vi "cDLTS measurement.vi"(5 "Session properties":T2, 7 "Workspace":path, 8 "Error In":errorcluster, 9 "myDLTS file path":path=path "", 10 "cDLTS measurement":T22={"Name"="", "Comment"="", "Time"=timestamp(0 s since 1904-01-01), "Folder"=path "", "DLTS properties"={"Tstart"=100.0, "Instant start"=FALSE, "Tstop"=350.0, "T rate"=0.016666666666666666, "Test signal"=0.1, "Test frequency"=100000.0, "Bandwidth"=0.0, "Averaging"=5.0, "Vbias"=-5.0, "Vpulse"=-1.0, "pulse length"=0.1, "Pulse 2"=FALSE, "Vpulse 2"=0.0, "pulse length 2"=0.0, "I range"=-2.0, "V range"=10.0, "Emission rate"=[10.0], "Sampling rate"=107000.0, "Acq. delay"=0.0, "Filter order"=0, "Equivalent circuit model"=0}, "GUID"=""} {"DLTS properties"."Equivalent circuit model" items=["Rp || Cp", "Rs + Cs", "Rs + Ls", "G B", "D Cs", "Q Cs", "D Ls", "Q Ls", "Rp || Lp", "D Cp"]; "DLTS properties"."Filter order" min=0 max=8 step=1; "DLTS properties"."Sampling rate" items=["13k"=13392.857422, "27k"=26785.714844, "54k"=53571.429687, "107k"=107142.859375]; "DLTS properties"."V range" items=["10mV"=0.01, "100mV"=0.1, "1V"=1.0, "10V"=10.0]; "DLTS properties"."I range" items=["10mV"=0.01, "100mV"=0.1, "1V"=1.0, "10V"=10.0]}, 11 "Loop data":T3={"Persistent"={"Last file"=path "", "Last user"="", "Users"=[]}, "Temp handle"={"Connected"=FALSE, "Temp ctrl"={"Gain (P)"=0.0, "Reset (I)"=0.0, "Rate (D)"=0.0, "Stabilization rate"=0.0, "Stabilization delta"=0.0, "Type"=enum."Lake Shore 325", "Custom temp ctrl"={"VISA resource name"=""}, "Lakeshore 325"={"VISA name"="", "Loop"=0, "Heater Range"=1, "Heater Resistance"=0, "Sample sensor"=0, "Fast sensor"=0, "Slow sensor"=0}, "Lakeshore 331"={"VISA name"="", "Loop"=1, "Heater Range"=0, "Sample sensor"=0, "Fast sensor"=0, "Slow sensor"=0}, "Lakeshore 332"={"VISA name"="", "Loop"=1, "Heater Range"=0, "Sample sensor"=0, "Fast sensor"=0, "Slow sensor"=0}, "Lakeshore 335"={"VISA name"="", "Loop"=1, "Sample sensor"=0, "Fast sensor"=0, "Slow sensor"=0, "Heater Range"=0, "Output mode"=enum."Off"}, "Lakeshore 336"={"VISA name"="", "Loop"=1, "Output mode"=enum."Off", "Max current"=1.0, "Heater resistance"=1, "Sample sensor"=1, "Slow sensor"=1, "Fast sensor"=1}}}, "Paths"={"Manual"=path "", "Settings"=path "", "Persistent"=path "", "Work dir."=path ""}, "Settings"={"MFIA"={"Address"="", "Use compensation"=TRUE, "Shut down gracefully"=FALSE}, "Temp ctrl"={"Gain (P)"=0.0, "Reset (I)"=0.0, "Rate (D)"=0.0, "Stabilization rate"=0.0, "Stabilization delta"=0.0, "Type"=enum."Lake Shore 325", "Custom temp ctrl"={"VISA resource name"=""}, "Lakeshore 325"={"VISA name"="", "Loop"=0, "Heater Range"=1, "Heater Resistance"=0, "Sample sensor"=0, "Fast sensor"=0, "Slow sensor"=0}, "Lakeshore 331"={"VISA name"="", "Loop"=1, "Heater Range"=0, "Sample sensor"=0, "Fast sensor"=0, "Slow sensor"=0}, "Lakeshore 332"={"VISA name"="", "Loop"=1, "Heater Range"=0, "Sample sensor"=0, "Fast sensor"=0, "Slow sensor"=0}, "Lakeshore 335"={"VISA name"="", "Loop"=1, "Sample sensor"=0, "Fast sensor"=0, "Slow sensor"=0, "Heater Range"=0, "Output mode"=enum."Off"}, "Lakeshore 336"={"VISA name"="", "Loop"=1, "Output mode"=enum."Off", "Max current"=1.0, "Heater resistance"=1, "Sample sensor"=1, "Slow sensor"=1, "Fast sensor"=1}}, "Source-meter"={"Type"=enum."Custom", "Custom source-meter"={"VISA resource name"=""}, "Keithley 2600"={"VISA name"="", "Ignore ID Query"=FALSE, "SMU"=enum."Channel A"}, "Keithley 2400 Series"={"VISA name"="", "Ignore ID Query"=FALSE}}, "Other"={"Enable OriginLab"=FALSE, "Reader mode"=FALSE, "Auto-save"=FALSE}, "Defaults"={"IV properties"={"T"=0.0, "Vstart"=-0.5, "Vstop"=0.5, "Vpoints"=10.0, "Settling"=0.01, "I limit"=0.1, "Log mapping"=FALSE, "Averaging"=0.0}, "CV properties"={"T"=0.0, "Vstart"=-0.5, "Vstop"=0.5, "Vpoints"=10.0, "Precision"=enum."Normal", "Test signal"=0.01, "Auto I range"=FALSE, "Test frequency"=100000.0, "I range"=-2.0, "V range"=10.0, "Log mapping"=FALSE, "Rel perm"=0.0, "Area"=0.0, "Equivalent circuit model"=0}, "DLTS properties"={"Tstart"=0.0, "Instant start"=FALSE, "Tstop"=0.0, "T rate"=0.0, "Test signal"=0.0, "Test frequency"=0.0, "Bandwidth"=0.0, "Averaging"=0.0, "Vbias"=0.0, "Vpulse"=0.0, "pulse length"=0.0, "Pulse 2"=FALSE, "Vpulse 2"=0.0, "pulse length 2"=0.0, "I range"=-2.0, "V range"=10.0, "Emission rate"=[], "Sampling rate"=0.0, "Acq. delay"=0.0, "Filter order"=0, "Equivalent circuit model"=0}, "LDLTS properties"={"T"=0.0, "Test signal"=0.0, "Test frequency"=0.0, "Bandwidth"=0.0, "Averaging"=0.0, "Vbias"=0.0, "Vpulse"=0.0, "pulse length"=0.0, "Pulse 2"=FALSE, "Vpulse 2"=0.0, "pulse length 2"=0.0, "I range"=-2.0, "V range"=10.0, "Sampling rate"=0.0, "Acq. delay"=0.0, "Sampling time"=0.0, "Filter order"=0, "Equivalent circuit model"=0}}}, "Software version"=0.0, "MFIA handle"={"ziHandle"={"handleValid"=FALSE, "Conn"=0, "Path Prefix"="", "Handle"=0, "Connected"=FALSE, "Clockbase(s)"=0.0}, "Selected device"="", "ziModHandle"={"handleValid"=FALSE, "Conn"=0, "ModHandle"=0, "moduleID"="", "Path Prefix"=""}}, "Source-meter handle"={"Connected"=FALSE, "Source-meter"={"Type"=enum."Custom", "Custom source-meter"={"VISA resource name"=""}, "Keithley 2600"={"VISA name"="", "Ignore ID Query"=FALSE, "SMU"=enum."Channel A"}, "Keithley 2400 Series"={"VISA name"="", "Ignore ID Query"=FALSE}}}} {"MFIA handle"."ziModHandle"."ModHandle" format="0x%08x"; "MFIA handle"."ziModHandle"."Conn" format="0x%08x"; "MFIA handle"."ziHandle"."Handle" format="0x%08x"; "MFIA handle"."ziHandle"."Conn" format="0x%08x"; "Settings"."Defaults"."LDLTS properties"."Equivalent circuit model" items=["Rp || Cp", "Rs + Cs", "Rs + Ls", "G B", "D Cs", "Q Cs", "D Ls", "Q Ls", "Rp || Lp", "D Cp"]; "Settings"."Defaults"."LDLTS properties"."Filter order" min=0 max=8 step=1; "Settings"."Defaults"."LDLTS properties"."Sampling rate" items=["13k"=13392.857422, "27k"=26785.714844, "54k"=53571.429687, "107k"=107142.859375]; "Settings"."Defaults"."LDLTS properties"."V range" items=["10mV"=0.01, "100mV"=0.1, "1V"=1.0, "10V"=10.0]; "Settings"."Defaults"."LDLTS properties"."I range" items=["100nA"=-7.0, "1µA"=-6.0, "10µA"=-5.0, "100µA"=-4.0, "1mA"=-3.0, "10mA"=-2.0]; "Settings"."Defaults"."DLTS properties"."Equivalent circuit model" items=["Rp || Cp", "Rs + Cs", "Rs + Ls", "G B", "D Cs", "Q Cs", "D Ls", "Q Ls", "Rp || Lp", "D Cp"]; "Settings"."Defaults"."DLTS properties"."Filter order" min=0 max=8 step=1; "Settings"."Defaults"."DLTS properties"."Sampling rate" items=["13k"=13392.857422, "27k"=26785.714844, "54k"=53571.429687, "107k"=107142.859375]; "Settings"."Defaults"."DLTS properties"."V range" items=["10mV"=0.01, "100mV"=0.1, "1V"=1.0, "10V"=10.0]; "Settings"."Defaults"."DLTS properties"."I range" items=["10mV"=0.01, "100mV"=0.1, "1V"=1.0, "10V"=10.0]; "Settings"."Defaults"."CV properties"."Equivalent circuit model" items=["Rp || Cp", "Rs + Cs", "Rs + Ls", "G B", "D Cs", "Q Cs", "D Ls", "Q Ls", "Rp || Lp", "D Cp"]; "Settings"."Defaults"."CV properties"."V range" items=["10mV"=0.01, "100mV"=0.1, "1V"=1.0, "10V"=10.0]; "Settings"."Defaults"."CV properties"."I range" items=["100nA"=-7.0, "1µA"=-6.0, "10µA"=-5.0, "100µA"=-4.0, "1mA"=-3.0, "10mA"=-2.0]; "Settings"."Defaults"."IV properties"."Settling" min=0.0 max=65535.0; "Settings"."Temp ctrl"."Lakeshore 336"."Fast sensor" items=["Sensor A", "Sensor B", "Sensor C", "Sensor D"]; "Settings"."Temp ctrl"."Lakeshore 336"."Slow sensor" items=["Sensor A", "Sensor B", "Sensor C", "Sensor D"]; "Settings"."Temp ctrl"."Lakeshore 336"."Sample sensor" items=["Sensor A", "Sensor B", "Sensor C", "Sensor D"]; "Settings"."Temp ctrl"."Lakeshore 336"."Heater resistance" items=["25 Ohm"=1, "50 Ohm"=2]; "Settings"."Temp ctrl"."Lakeshore 336"."Max current" items=["0.707 A"=0.0, "1 A"=1.0, "1.414 A"=1.414, "2 A"=2.0]; "Settings"."Temp ctrl"."Lakeshore 336"."Loop" items=["Output 1"=1, "Output 2"=2, "Output 3"=3, "Output 4"=4]; "Settings"."Temp ctrl"."Lakeshore 335"."Heater Range" items=["Off", "Low (On)", "Medium", "High"]; "Settings"."Temp ctrl"."Lakeshore 335"."Slow sensor" items=["A", "B"]; "Settings"."Temp ctrl"."Lakeshore 335"."Fast sensor" items=["A", "B"]; "Settings"."Temp ctrl"."Lakeshore 335"."Sample sensor" items=["A", "B"]; "Settings"."Temp ctrl"."Lakeshore 335"."Loop" items=["Loop 1"=1, "Loop 2"=2]; "Settings"."Temp ctrl"."Lakeshore 332"."Slow sensor" items=["A", "B"]; "Settings"."Temp ctrl"."Lakeshore 332"."Fast sensor" items=["A", "B"]; "Settings"."Temp ctrl"."Lakeshore 332"."Sample sensor" items=["A", "B"]; "Settings"."Temp ctrl"."Lakeshore 332"."Heater Range" items=["Off", "Low (0.5W)", "Med (5W)", "High (50W)"]; "Settings"."Temp ctrl"."Lakeshore 332"."Loop" items=["Loop 1", "Loop 2"]; "Settings"."Temp ctrl"."Lakeshore 331"."Slow sensor" items=["A", "B"]; "Settings"."Temp ctrl"."Lakeshore 331"."Fast sensor" items=["A", "B"]; "Settings"."Temp ctrl"."Lakeshore 331"."Sample sensor" items=["A", "B"]; "Settings"."Temp ctrl"."Lakeshore 331"."Heater Range" items=["Off", "Low (0.5W)", "Med (5W)", "High (50W)"]; "Settings"."Temp ctrl"."Lakeshore 331"."Loop" items=["Loop 1", "Loop 2"]; "Settings"."Temp ctrl"."Lakeshore 325"."Slow sensor" items=["A", "B"]; "Settings"."Temp ctrl"."Lakeshore 325"."Fast sensor" items=["A", "B"]; "Settings"."Temp ctrl"."Lakeshore 325"."Sample sensor" items=["A", "B"]; "Settings"."Temp ctrl"."Lakeshore 325"."Heater Resistance" items=["25 Ohm"=1, "50 Ohm"=2]; "Settings"."Temp ctrl"."Lakeshore 325"."Heater Range" items=["Off", "Low (loop 1) or On (loop 2)", "High (loop 1)"]; "Settings"."Temp ctrl"."Lakeshore 325"."Loop" items=["Loop 1"=1, "Loop 2"=2]; "Temp handle"."Temp ctrl"."Lakeshore 336"."Fast sensor" items=["Sensor A", "Sensor B", "Sensor C", "Sensor D"]; "Temp handle"."Temp ctrl"."Lakeshore 336"."Slow sensor" items=["Sensor A", "Sensor B", "Sensor C", "Sensor D"]; "Temp handle"."Temp ctrl"."Lakeshore 336"."Sample sensor" items=["Sensor A", "Sensor B", "Sensor C", "Sensor D"]; "Temp handle"."Temp ctrl"."Lakeshore 336"."Heater resistance" items=["25 Ohm"=1, "50 Ohm"=2]; "Temp handle"."Temp ctrl"."Lakeshore 336"."Max current" items=["0.707 A"=0.0, "1 A"=1.0, "1.414 A"=1.414, "2 A"=2.0]; "Temp handle"."Temp ctrl"."Lakeshore 336"."Loop" items=["Output 1"=1, "Output 2"=2, "Output 3"=3, "Output 4"=4]; "Temp handle"."Temp ctrl"."Lakeshore 335"."Heater Range" items=["Off", "Low (On)", "Medium", "High"]; "Temp handle"."Temp ctrl"."Lakeshore 335"."Slow sensor" items=["A", "B"]; "Temp handle"."Temp ctrl"."Lakeshore 335"."Fast sensor" items=["A", "B"]; "Temp handle"."Temp ctrl"."Lakeshore 335"."Sample sensor" items=["A", "B"]; "Temp handle"."Temp ctrl"."Lakeshore 335"."Loop" items=["Loop 1"=1, "Loop 2"=2]; "Temp handle"."Temp ctrl"."Lakeshore 332"."Slow sensor" items=["A", "B"]; "Temp handle"."Temp ctrl"."Lakeshore 332"."Fast sensor" items=["A", "B"]; "Temp handle"."Temp ctrl"."Lakeshore 332"."Sample sensor" items=["A", "B"]; "Temp handle"."Temp ctrl"."Lakeshore 332"."Heater Range" items=["Off", "Low (0.5W)", "Med (5W)", "High (50W)"]; "Temp handle"."Temp ctrl"."Lakeshore 332"."Loop" items=["Loop 1", "Loop 2"]; "Temp handle"."Temp ctrl"."Lakeshore 331"."Slow sensor" items=["A", "B"]; "Temp handle"."Temp ctrl"."Lakeshore 331"."Fast sensor" items=["A", "B"]; "Temp handle"."Temp ctrl"."Lakeshore 331"."Sample sensor" items=["A", "B"]; "Temp handle"."Temp ctrl"."Lakeshore 331"."Heater Range" items=["Off", "Low (0.5W)", "Med (5W)", "High (50W)"]; "Temp handle"."Temp ctrl"."Lakeshore 331"."Loop" items=["Loop 1", "Loop 2"]; "Temp handle"."Temp ctrl"."Lakeshore 325"."Slow sensor" items=["A", "B"]; "Temp handle"."Temp ctrl"."Lakeshore 325"."Fast sensor" items=["A", "B"]; "Temp handle"."Temp ctrl"."Lakeshore 325"."Sample sensor" items=["A", "B"]; "Temp handle"."Temp ctrl"."Lakeshore 325"."Heater Resistance" items=["25 Ohm"=1, "50 Ohm"=2]; "Temp handle"."Temp ctrl"."Lakeshore 325"."Heater Range" items=["Off", "Low (loop 1) or On (loop 2)", "High (loop 1)"]; "Temp handle"."Temp ctrl"."Lakeshore 325"."Loop" items=["Loop 1"=1, "Loop 2"=2]}) -> (0 "Error Out":errorcluster, 1 "Modified":bool, 2 "cDLTS measurement out":T22={"Name"="", "Comment"="", "Time"=timestamp(0 s since 1904-01-01), "Folder"=path "", "DLTS properties"={"Tstart"=0.0, "Instant start"=FALSE, "Tstop"=0.0, "T rate"=0.0, "Test signal"=0.0, "Test frequency"=0.0, "Bandwidth"=0.0, "Averaging"=0.0, "Vbias"=0.0, "Vpulse"=0.0, "pulse length"=0.0, "Pulse 2"=FALSE, "Vpulse 2"=0.0, "pulse length 2"=0.0, "I range"=-2.0, "V range"=10.0, "Emission rate"=[], "Sampling rate"=0.0, "Acq. delay"=0.0, "Filter order"=0, "Equivalent circuit model"=0}, "GUID"=""} {"DLTS properties"."Equivalent circuit model" items=["Rp || Cp", "Rs + Cs", "Rs + Ls", "G B", "D Cs", "Q Cs", "D Ls", "Q Ls", "Rp || Lp", "D Cp"]; "DLTS properties"."Filter order" min=0 max=8 step=1; "DLTS properties"."Sampling rate" items=["13k"=13392.857422, "27k"=26785.714844, "54k"=53571.429687, "107k"=107142.859375]; "DLTS properties"."V range" items=["10mV"=0.01, "100mV"=0.1, "1V"=1.0, "10V"=10.0]; "DLTS properties"."I range" items=["10mV"=0.01, "100mV"=0.1, "1V"=1.0, "10V"=10.0]}, 3 "Loop data out":T3={"Persistent"={"Last file"=path "", "Last user"="", "Users"=[]}, "Temp handle"={"Connected"=FALSE, "Temp ctrl"={"Gain (P)"=0.0, "Reset (I)"=0.0, "Rate (D)"=0.0, "Stabilization rate"=0.0, "Stabilization delta"=0.0, "Type"=enum."Lake Shore 325", "Custom temp ctrl"={"VISA resource name"=""}, "Lakeshore 325"={"VISA name"="", "Loop"=0, "Heater Range"=1, "Heater Resistance"=0, "Sample sensor"=0, "Fast sensor"=0, "Slow sensor"=0}, "Lakeshore 331"={"VISA name"="", "Loop"=1, "Heater Range"=0, "Sample sensor"=0, "Fast sensor"=0, "Slow sensor"=0}, "Lakeshore 332"={"VISA name"="", "Loop"=1, "Heater Range"=0, "Sample sensor"=0, "Fast sensor"=0, "Slow sensor"=0}, "Lakeshore 335"={"VISA name"="", "Loop"=1, "Sample sensor"=0, "Fast sensor"=0, "Slow sensor"=0, "Heater Range"=0, "Output mode"=enum."Off"}, "Lakeshore 336"={"VISA name"="", "Loop"=1, "Output mode"=enum."Off", "Max current"=1.0, "Heater resistance"=1, "Sample sensor"=1, "Slow sensor"=1, "Fast sensor"=1}}}, "Paths"={"Manual"=path "", "Settings"=path "", "Persistent"=path "", "Work dir."=path ""}, "Settings"={"MFIA"={"Address"="", "Use compensation"=TRUE, "Shut down gracefully"=FALSE}, "Temp ctrl"={"Gain (P)"=0.0, "Reset (I)"=0.0, "Rate (D)"=0.0, "Stabilization rate"=0.0, "Stabilization delta"=0.0, "Type"=enum."Lake Shore 325", "Custom temp ctrl"={"VISA resource name"=""}, "Lakeshore 325"={"VISA name"="", "Loop"=0, "Heater Range"=1, "Heater Resistance"=0, "Sample sensor"=0, "Fast sensor"=0, "Slow sensor"=0}, "Lakeshore 331"={"VISA name"="", "Loop"=1, "Heater Range"=0, "Sample sensor"=0, "Fast sensor"=0, "Slow sensor"=0}, "Lakeshore 332"={"VISA name"="", "Loop"=1, "Heater Range"=0, "Sample sensor"=0, "Fast sensor"=0, "Slow sensor"=0}, "Lakeshore 335"={"VISA name"="", "Loop"=1, "Sample sensor"=0, "Fast sensor"=0, "Slow sensor"=0, "Heater Range"=0, "Output mode"=enum."Off"}, "Lakeshore 336"={"VISA name"="", "Loop"=1, "Output mode"=enum."Off", "Max current"=1.0, "Heater resistance"=1, "Sample sensor"=1, "Slow sensor"=1, "Fast sensor"=1}}, "Source-meter"={"Type"=enum."Custom", "Custom source-meter"={"VISA resource name"=""}, "Keithley 2600"={"VISA name"="", "Ignore ID Query"=FALSE, "SMU"=enum."Channel A"}, "Keithley 2400 Series"={"VISA name"="", "Ignore ID Query"=FALSE}}, "Other"={"Enable OriginLab"=FALSE, "Reader mode"=FALSE, "Auto-save"=FALSE}, "Defaults"={"IV properties"={"T"=0.0, "Vstart"=-0.5, "Vstop"=0.5, "Vpoints"=10.0, "Settling"=0.01, "I limit"=0.1, "Log mapping"=FALSE, "Averaging"=0.0}, "CV properties"={"T"=0.0, "Vstart"=-0.5, "Vstop"=0.5, "Vpoints"=10.0, "Precision"=enum."Normal", "Test signal"=0.01, "Auto I range"=FALSE, "Test frequency"=100000.0, "I range"=-2.0, "V range"=10.0, "Log mapping"=FALSE, "Rel perm"=0.0, "Area"=0.0, "Equivalent circuit model"=0}, "DLTS properties"={"Tstart"=0.0, "Instant start"=FALSE, "Tstop"=0.0, "T rate"=0.0, "Test signal"=0.0, "Test frequency"=0.0, "Bandwidth"=0.0, "Averaging"=0.0, "Vbias"=0.0, "Vpulse"=0.0, "pulse length"=0.0, "Pulse 2"=FALSE, "Vpulse 2"=0.0, "pulse length 2"=0.0, "I range"=-2.0, "V range"=10.0, "Emission rate"=[], "Sampling rate"=0.0, "Acq. delay"=0.0, "Filter order"=0, "Equivalent circuit model"=0}, "LDLTS properties"={"T"=0.0, "Test signal"=0.0, "Test frequency"=0.0, "Bandwidth"=0.0, "Averaging"=0.0, "Vbias"=0.0, "Vpulse"=0.0, "pulse length"=0.0, "Pulse 2"=FALSE, "Vpulse 2"=0.0, "pulse length 2"=0.0, "I range"=-2.0, "V range"=10.0, "Sampling rate"=0.0, "Acq. delay"=0.0, "Sampling time"=0.0, "Filter order"=0, "Equivalent circuit model"=0}}}, "Software version"=0.0, "MFIA handle"={"ziHandle"={"handleValid"=FALSE, "Conn"=0, "Path Prefix"="", "Handle"=0, "Connected"=FALSE, "Clockbase(s)"=0.0}, "Selected device"="", "ziModHandle"={"handleValid"=FALSE, "Conn"=0, "ModHandle"=0, "moduleID"="", "Path Prefix"=""}}, "Source-meter handle"={"Connected"=FALSE, "Source-meter"={"Type"=enum."Custom", "Custom source-meter"={"VISA resource name"=""}, "Keithley 2600"={"VISA name"="", "Ignore ID Query"=FALSE, "SMU"=enum."Channel A"}, "Keithley 2400 Series"={"VISA name"="", "Ignore ID Query"=FALSE}}}} {"MFIA handle"."ziModHandle"."ModHandle" format="0x%08x"; "MFIA handle"."ziModHandle"."Conn" format="0x%08x"; "MFIA handle"."ziHandle"."Handle" format="0x%08x"; "MFIA handle"."ziHandle"."Conn" format="0x%08x"; "Settings"."Defaults"."LDLTS properties"."Equivalent circuit model" items=["Rp || Cp", "Rs + Cs", "Rs + Ls", "G B", "D Cs", "Q Cs", "D Ls", "Q Ls", "Rp || Lp", "D Cp"]; "Settings"."Defaults"."LDLTS properties"."Filter order" min=0 max=8 step=1; "Settings"."Defaults"."LDLTS properties"."Sampling rate" items=["13k"=13392.857422, "27k"=26785.714844, "54k"=53571.429687, "107k"=107142.859375]; "Settings"."Defaults"."LDLTS properties"."V range" items=["10mV"=0.01, "100mV"=0.1, "1V"=1.0, "10V"=10.0]; "Settings"."Defaults"."LDLTS properties"."I range" items=["100nA"=-7.0, "1µA"=-6.0, "10µA"=-5.0, "100µA"=-4.0, "1mA"=-3.0, "10mA"=-2.0]; "Settings"."Defaults"."DLTS properties"."Equivalent circuit model" items=["Rp || Cp", "Rs + Cs", "Rs + Ls", "G B", "D Cs", "Q Cs", "D Ls", "Q Ls", "Rp || Lp", "D Cp"]; "Settings"."Defaults"."DLTS properties"."Filter order" min=0 max=8 step=1; "Settings"."Defaults"."DLTS properties"."Sampling rate" items=["13k"=13392.857422, "27k"=26785.714844, "54k"=53571.429687, "107k"=107142.859375]; "Settings"."Defaults"."DLTS properties"."V range" items=["10mV"=0.01, "100mV"=0.1, "1V"=1.0, "10V"=10.0]; "Settings"."Defaults"."DLTS properties"."I range" items=["10mV"=0.01, "100mV"=0.1, "1V"=1.0, "10V"=10.0]; "Settings"."Defaults"."CV properties"."Equivalent circuit model" items=["Rp || Cp", "Rs + Cs", "Rs + Ls", "G B", "D Cs", "Q Cs", "D Ls", "Q Ls", "Rp || Lp", "D Cp"]; "Settings"."Defaults"."CV properties"."V range" items=["10mV"=0.01, "100mV"=0.1, "1V"=1.0, "10V"=10.0]; "Settings"."Defaults"."CV properties"."I range" items=["100nA"=-7.0, "1µA"=-6.0, "10µA"=-5.0, "100µA"=-4.0, "1mA"=-3.0, "10mA"=-2.0]; "Settings"."Defaults"."IV properties"."Settling" min=0.0 max=65535.0; "Settings"."Temp ctrl"."Lakeshore 336"."Fast sensor" items=["Sensor A", "Sensor B", "Sensor C", "Sensor D"]; "Settings"."Temp ctrl"."Lakeshore 336"."Slow sensor" items=["Sensor A", "Sensor B", "Sensor C", "Sensor D"]; "Settings"."Temp ctrl"."Lakeshore 336"."Sample sensor" items=["Sensor A", "Sensor B", "Sensor C", "Sensor D"]; "Settings"."Temp ctrl"."Lakeshore 336"."Heater resistance" items=["25 Ohm"=1, "50 Ohm"=2]; "Settings"."Temp ctrl"."Lakeshore 336"."Max current" items=["0.707 A"=0.0, "1 A"=1.0, "1.414 A"=1.414, "2 A"=2.0]; "Settings"."Temp ctrl"."Lakeshore 336"."Loop" items=["Output 1"=1, "Output 2"=2, "Output 3"=3, "Output 4"=4]; "Settings"."Temp ctrl"."Lakeshore 335"."Heater Range" items=["Off", "Low (On)", "Medium", "High"]; "Settings"."Temp ctrl"."Lakeshore 335"."Slow sensor" items=["A", "B"]; "Settings"."Temp ctrl"."Lakeshore 335"."Fast sensor" items=["A", "B"]; "Settings"."Temp ctrl"."Lakeshore 335"."Sample sensor" items=["A", "B"]; "Settings"."Temp ctrl"."Lakeshore 335"."Loop" items=["Loop 1"=1, "Loop 2"=2]; "Settings"."Temp ctrl"."Lakeshore 332"."Slow sensor" items=["A", "B"]; "Settings"."Temp ctrl"."Lakeshore 332"."Fast sensor" items=["A", "B"]; "Settings"."Temp ctrl"."Lakeshore 332"."Sample sensor" items=["A", "B"]; "Settings"."Temp ctrl"."Lakeshore 332"."Heater Range" items=["Off", "Low (0.5W)", "Med (5W)", "High (50W)"]; "Settings"."Temp ctrl"."Lakeshore 332"."Loop" items=["Loop 1", "Loop 2"]; "Settings"."Temp ctrl"."Lakeshore 331"."Slow sensor" items=["A", "B"]; "Settings"."Temp ctrl"."Lakeshore 331"."Fast sensor" items=["A", "B"]; "Settings"."Temp ctrl"."Lakeshore 331"."Sample sensor" items=["A", "B"]; "Settings"."Temp ctrl"."Lakeshore 331"."Heater Range" items=["Off", "Low (0.5W)", "Med (5W)", "High (50W)"]; "Settings"."Temp ctrl"."Lakeshore 331"."Loop" items=["Loop 1", "Loop 2"]; "Settings"."Temp ctrl"."Lakeshore 325"."Slow sensor" items=["A", "B"]; "Settings"."Temp ctrl"."Lakeshore 325"."Fast sensor" items=["A", "B"]; "Settings"."Temp ctrl"."Lakeshore 325"."Sample sensor" items=["A", "B"]; "Settings"."Temp ctrl"."Lakeshore 325"."Heater Resistance" items=["25 Ohm"=1, "50 Ohm"=2]; "Settings"."Temp ctrl"."Lakeshore 325"."Heater Range" items=["Off", "Low (loop 1) or On (loop 2)", "High (loop 1)"]; "Settings"."Temp ctrl"."Lakeshore 325"."Loop" items=["Loop 1"=1, "Loop 2"=2]; "Temp handle"."Temp ctrl"."Lakeshore 336"."Fast sensor" items=["Sensor A", "Sensor B", "Sensor C", "Sensor D"]; "Temp handle"."Temp ctrl"."Lakeshore 336"."Slow sensor" items=["Sensor A", "Sensor B", "Sensor C", "Sensor D"]; "Temp handle"."Temp ctrl"."Lakeshore 336"."Sample sensor" items=["Sensor A", "Sensor B", "Sensor C", "Sensor D"]; "Temp handle"."Temp ctrl"."Lakeshore 336"."Heater resistance" items=["25 Ohm"=1, "50 Ohm"=2]; "Temp handle"."Temp ctrl"."Lakeshore 336"."Max current" items=["0.707 A"=0.0, "1 A"=1.0, "1.414 A"=1.414, "2 A"=2.0]; "Temp handle"."Temp ctrl"."Lakeshore 336"."Loop" items=["Output 1"=1, "Output 2"=2, "Output 3"=3, "Output 4"=4]; "Temp handle"."Temp ctrl"."Lakeshore 335"."Heater Range" items=["Off", "Low (On)", "Medium", "High"]; "Temp handle"."Temp ctrl"."Lakeshore 335"."Slow sensor" items=["A", "B"]; "Temp handle"."Temp ctrl"."Lakeshore 335"."Fast sensor" items=["A", "B"]; "Temp handle"."Temp ctrl"."Lakeshore 335"."Sample sensor" items=["A", "B"]; "Temp handle"."Temp ctrl"."Lakeshore 335"."Loop" items=["Loop 1"=1, "Loop 2"=2]; "Temp handle"."Temp ctrl"."Lakeshore 332"."Slow sensor" items=["A", "B"]; "Temp handle"."Temp ctrl"."Lakeshore 332"."Fast sensor" items=["A", "B"]; "Temp handle"."Temp ctrl"."Lakeshore 332"."Sample sensor" items=["A", "B"]; "Temp handle"."Temp ctrl"."Lakeshore 332"."Heater Range" items=["Off", "Low (0.5W)", "Med (5W)", "High (50W)"]; "Temp handle"."Temp ctrl"."Lakeshore 332"."Loop" items=["Loop 1", "Loop 2"]; "Temp handle"."Temp ctrl"."Lakeshore 331"."Slow sensor" items=["A", "B"]; "Temp handle"."Temp ctrl"."Lakeshore 331"."Fast sensor" items=["A", "B"]; "Temp handle"."Temp ctrl"."Lakeshore 331"."Sample sensor" items=["A", "B"]; "Temp handle"."Temp ctrl"."Lakeshore 331"."Heater Range" items=["Off", "Low (0.5W)", "Med (5W)", "High (50W)"]; "Temp handle"."Temp ctrl"."Lakeshore 331"."Loop" items=["Loop 1", "Loop 2"]; "Temp handle"."Temp ctrl"."Lakeshore 325"."Slow sensor" items=["A", "B"]; "Temp handle"."Temp ctrl"."Lakeshore 325"."Fast sensor" items=["A", "B"]; "Temp handle"."Temp ctrl"."Lakeshore 325"."Sample sensor" items=["A", "B"]; "Temp handle"."Temp ctrl"."Lakeshore 325"."Heater Resistance" items=["25 Ohm"=1, "50 Ohm"=2]; "Temp handle"."Temp ctrl"."Lakeshore 325"."Heater Range" items=["Off", "Low (loop 1) or On (loop 2)", "High (loop 1)"]; "Temp handle"."Temp ctrl"."Lakeshore 325"."Loop" items=["Loop 1"=1, "Loop 2"=2]})   [LabVIEW 2019]
doc: "Handles conventional DLTS measurement, displays cDLTS GUI window"
uses:
  Type defs/Loop data Type Def.ctl
  Type defs/Persistent Type Def.ctl
  Type defs/Temp handle Type Def.ctl
  Type defs/Temp ctrl Type Def.ctl
  Custom devices/Custom temp ctrl settings.ctl
  Type defs/Paths Type Def.ctl
  Type defs/Settings Type Def.ctl
  Type defs/Imps Type Def.ctl
  Type defs/Source-meter Type Def.ctl
  Custom devices/Custom source-meter settings.ctl
  Type defs/Other settings Type Def.ctl
  Type defs/IV properties Type Def.ctl
  Type defs/CV properties Type Def.ctl
  Type defs/DLTS properties Type Def.ctl
  Type defs/LDLTS properties Type Def.ctl
  Type defs/MFIA handle Type Def.ctl
  <instrlib>/Zurich Instruments LabOne/Public/ziTypeHandle.ctl
  <instrlib>/Zurich Instruments LabOne/Public/Modules/ziTypeModHandle.ctl
  Type defs/Source-meter handle Type Def.ctl
  Type defs/cDLTS measurement Type Def.ctl
  Type defs/Session properties Type Def.ctl
  <vilib>/Utility/miscctls.llb/LVPointTypeDef.ctl
  <vilib>/Utility/error.llb/DialogType.ctl
  <vilib>/TaskbarProgressAPI/_TypeDefs/Progress State.ctl
  DLTS - timing calculation (time window) (SubVI).vi
  <instrlib>/Zurich Instruments LabOne/Public/Configure/ziSetValueDouble.vi
  Export single clipboard - cDLTS cluster.vi
  Export single dat - cDLTS cluster.vi
  Export Origin - cDLTS.vi
  DLTS - timing calculation (emission rates) (SubVI).vi
  <instrlib>/Zurich Instruments LabOne/Zurich Instruments LabOne.lvlib
  <vilib>/TaskbarProgressAPI/TaskbarProgressAPI.lvlib
panel:
  in  "Model":u16(ring) caption="Equivalent circuit model" items=["Rp || Cp", "Rs + Cs"]
  in  "Filter order":i32=8 caption="Numeric" min=1 max=8 step=1
  out "Filter rise time":dbl[unit]=10.0 caption="Numeric" min=0.1 max=100.0 format="%#_2p"
  in  "Folder":path
  in  "Enable post meas. T":bool caption="Enable"
  in  "Post meas. temp.":dbl[unit]=300.0 caption="Numeric" min=1.0 max=800.0 format="%#.0f"
  in  "Acquisition delay":dbl[unit]=1.0 caption="Numeric" min=0.0 max=1.0 step=1e-06 format="%#_6p"
  in  "2nd pulse":bool=TRUE caption="2 pulse mode:"
  in  "2nd pulse length":dbl[unit]=100.0 caption="2nd pulse duration" min=1e-06 max=100.0 format="%#_6p"
  in  "2nd pulse voltage":dbl[unit]=0.01 caption="Numeric" min=-10.0 max=10.0 format="%#_6p"
  in  "Sampling rate":dbl(ring)=107142.859375 caption="Ring" items=["13 kSa"=13392.857422, "27 kSa"=26785.714844, "54 kSa"=53571.429687, "107 kSa"=107142.859375]
  in  "Filter bandwidth":dbl[unit]=10000.0 caption="Numeric" min=100.0 max=100000.0 format="%#_6p"
  in  "Stop":bool
  out "Single transient capture duration":dbl[unit] caption="Numeric" format="%#.1p"
  out "No samples":dbl caption="Number of samples per transient" format="%#.0f"
  in  "Rate windows":dbl[unit][](array[numeric]) min=1.0 max=5000.0
  in  "Averaging":dbl=1.0 caption="Numeric" min=1.0 max=300.0 step=1.0
  in  "1st pulse length":dbl[unit]=100.0 caption="1st pulse duration" min=2.333e-07 max=1.0 format="%#.1p"
  in  "1st pulse voltage":dbl[unit]=0.01 caption="Numeric" min=-10.0 max=10.0 format="%#_6p"
  in  "Bias voltage":dbl[unit]=0.01 caption="Numeric" min=-10.0 max=10.0 format="%#_6p"
  in  "T rate":dbl[unit]=1.6666666666666667e-05 caption="Temperature change rate" min=1.6666666666666667e-05 max=1.6666666666666667 format="%#.1g"
  in  "Instant T start":bool=TRUE caption="Instant"
  in  "Stop temp.":dbl[unit]=1.0 caption="Numeric" min=1.0 max=800.0
  in  "Start temp.":dbl[unit]=1.0 caption="Numeric" min=1.0 max=800.0 format="%#.0f"
  in  "V range":dbl[unit](ring)=10.0 caption="Voltage range" items=["10mV"=0.01, "100mV"=0.1, "1V"=1.0, "10V"=10.0]
  in  "Test frequency":dbl[unit]=100000.0 caption="Numeric" min=10000.0 max=5000000000.0 format="%#_6p"
  in  "I range":dbl(ring)=-7.0 caption="Current range" items=["100nA"=-7.0, "1µA"=-6.0, "10µA"=-5.0, "100µA"=-4.0, "1mA"=-3.0, "10mA"=-2.0]
  in  "Measure":bool
  in  "Test signal":dbl[unit]=0.3 caption="Numeric" min=1e-06 max=1.0 format="%#_6p"
  in  "Setpoint":dbl[unit]=1.0 caption="Numeric" min=1.0 max=800.0
  out "Temperature":dbl[unit] caption="Numeric"
  out "Measurement info":string
  in  "Top Buttons":T1
  out "DLTS Signal Graph":cluster{"2D data":dbl[], "2D data":dbl[]}[](graph)
  out "Transient Graph":cluster{"t":dbl[], "Samples":dbl[]}(graph)
  out "Temp Chart":dbl(graph)=189.08
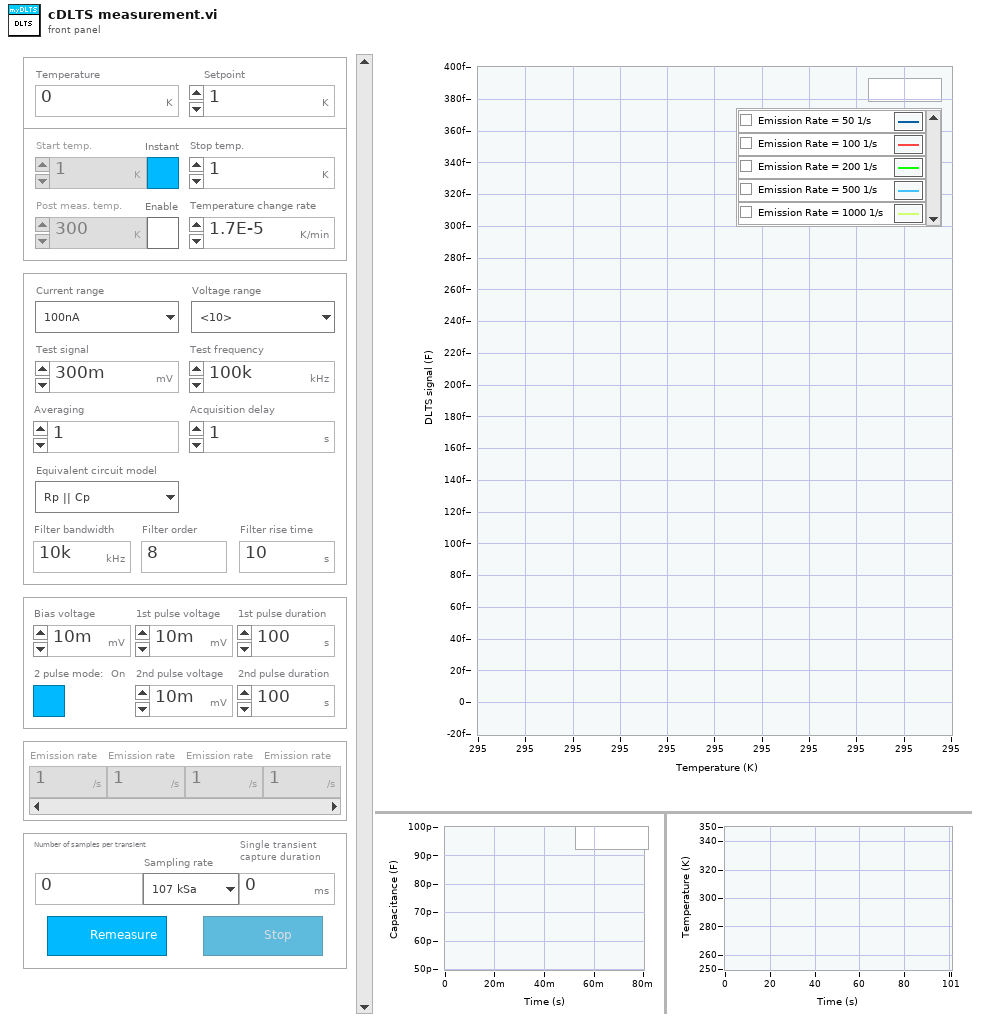
[diagram p1: front panel]
types:
  T1 = cluster{"Information":bool, "Help":bool, "Save Parameters":bool, "Export":bool}
  T2 = typedef "Session properties Type Def.ctl" = cluster{"Session name":string, "Comment":string, "User":string, "Software version":dbl, "Created":timestamp, "Modified":timestamp, "Binary":bool, "GUID":string}
  T3 = typedef "Loop data Type Def.ctl" = cluster{"Persistent":T4, "Temp handle":T5, "Paths":T8, "Settings":T9, "Software version":dbl, "MFIA handle":T18, "Source-meter handle":T21}
  T4 = typedef "Persistent Type Def.ctl" = cluster{"Last file":path, "Last user":string, "Users":cluster{"User":string, "Authors directory":path}[]}
  T5 = typedef "Temp handle Type Def.ctl" = cluster{"Connected":bool, "Temp ctrl":T6}
  T6 = typedef "Temp ctrl Type Def.ctl" = cluster{"Gain (P)":dbl, "Reset (I)":dbl, "Rate (D)":dbl, "Stabilization rate":dbl, "Stabilization delta":dbl, "Type":enum16{"Custom", "Lake Shore 325", "Lake Shore 331", "Lake Shore 332", "Lake Shore 335", "Lake Shore 336"}, "Custom temp ctrl":T7, "Lakeshore 325":cluster{"VISA name":refnum<visa-resource-name>, "Loop":u16, "Heater Range":u16, "Heater Resistance":u16, "Sample sensor":u16, "Fast sensor":u16, "Slow sensor":u16}, "Lakeshore 331":cluster{"VISA name":refnum<visa-resource-name>, "Loop":u16, "Heater Range":u16, "Sample sensor":u16, "Fast sensor":u16, "Slow sensor":u16}, "Lakeshore 332":cluster{"VISA name":refnum<visa-resource-name>, "Loop":u16, "Heater Range":u16, "Sample sensor":u16, "Fast sensor":u16, "Slow sensor":u16}, "Lakeshore 335":cluster{"VISA name":refnum<visa-resource-name>, "Loop":u16, "Sample sensor":u16, "Fast sensor":u16, "Slow sensor":u16, "Heater Range":u16, "Output mode":enum16{"Off", "Closed Loop PID", "Zone", "Open Loop", "Monitor Out", "Warmup Supply"}}, "Lakeshore 336":cluster{"VISA name":refnum<visa-resource-name>, "Loop":u16, "Output mode":enum16{"Off", "Closed Loop PID", "Zone", "Open Loop"}, "Max current":dbl, "Heater resistance":u16, "Sample sensor":u16, "Slow sensor":u16, "Fast sensor":u16}}
  T7 = typedef "Custom temp ctrl settings.ctl" = cluster{"VISA resource name":refnum<visa-resource-name>}
  T8 = typedef "Paths Type Def.ctl" = cluster{"Manual":path, "Settings":path, "Persistent":path, "Work dir.":path}
  T9 = typedef "Settings Type Def.ctl" = cluster{"MFIA":T10, "Temp ctrl":T6, "Source-meter":T11, "Other":T13, "Defaults":cluster{"IV properties":T14, "CV properties":T15, "DLTS properties":T16, "LDLTS properties":T17}}
  T10 = typedef "Imps Type Def.ctl" = cluster{"Address":string, "Use compensation":bool, "Shut down gracefully":bool}
  T11 = typedef "Source-meter Type Def.ctl" = cluster{"Type":enum16{"Custom", "Keithley 2600", "Keithley 2400 Series"}, "Custom source-meter":T12, "Keithley 2600":cluster{"VISA name":refnum<visa-resource-name>, "Ignore ID Query":bool, "SMU":enum16{"Channel A", "Channel B"}}, "Keithley 2400 Series":cluster{"VISA name":refnum<visa-resource-name>, "Ignore ID Query":bool}}
  T12 = typedef "Custom source-meter settings.ctl" = cluster{"VISA resource name":refnum<visa-resource-name>}
  T13 = typedef "Other settings Type Def.ctl" = cluster{"Enable OriginLab":bool, "Reader mode":bool, "Auto-save":bool}
  T14 = typedef "IV properties Type Def.ctl" = cluster{"T":dbl[unit], "Vstart":dbl[unit], "Vstop":dbl[unit], "Vpoints":dbl, "Settling":dbl[unit], "I limit":dbl[unit], "Log mapping":bool, "Averaging":dbl}
  T15 = typedef "CV properties Type Def.ctl" = cluster{"T":dbl[unit], "Vstart":dbl[unit], "Vstop":dbl[unit], "Vpoints":dbl, "Precision":enum16{"Low (Fast)", "Normal", "High (Slow)"}, "Test signal":dbl[unit], "Auto I range":bool, "Test frequency":dbl[unit], "I range":dbl, "V range":dbl[unit], "Log mapping":bool, "Rel perm":dbl, "Area":dbl[unit], "Equivalent circuit model":u16}
  T16 = typedef "DLTS properties Type Def.ctl" = cluster{"Tstart":dbl[unit], "Instant start":bool, "Tstop":dbl[unit], "T rate":dbl[unit], "Test signal":dbl[unit], "Test frequency":dbl[unit], "Bandwidth":dbl[unit], "Averaging":dbl, "Vbias":dbl[unit], "Vpulse":dbl[unit], "pulse length":dbl[unit], "Pulse 2":bool, "Vpulse 2":dbl[unit], "pulse length 2":dbl[unit], "I range":dbl, "V range":dbl[unit], "Emission rate":dbl[unit][], "Sampling rate":dbl[unit], "Acq. delay":dbl[unit], "Filter order":i32, "Equivalent circuit model":u16}
  T17 = typedef "LDLTS properties Type Def.ctl" = cluster{"T":dbl[unit], "Test signal":dbl[unit], "Test frequency":dbl[unit], "Bandwidth":dbl[unit], "Averaging":dbl, "Vbias":dbl[unit], "Vpulse":dbl[unit], "pulse length":dbl[unit], "Pulse 2":bool, "Vpulse 2":dbl[unit], "pulse length 2":dbl[unit], "I range":dbl, "V range":dbl[unit], "Sampling rate":dbl[unit], "Acq. delay":dbl[unit], "Sampling time":dbl[unit], "Filter order":i32, "Equivalent circuit model":u16}
  T18 = typedef "MFIA handle Type Def.ctl" = cluster{"ziHandle":T19, "Selected device":string, "ziModHandle":T20}
  T19 = typedef "Zurich Instruments LabOne.lvlib/ziTypeHandle.ctl" = cluster{"handleValid":bool, "Conn":u64, "Path Prefix":string, "Handle":u64, "Connected":bool, "Clockbase(s)":dbl}
  T20 = typedef "Zurich Instruments LabOne.lvlib/ziTypeModHandle.ctl" = cluster{"handleValid":bool, "Conn":u64, "ModHandle":u64, "moduleID":string, "Path Prefix":string}
  T21 = typedef "Source-meter handle Type Def.ctl" = cluster{"Connected":bool, "Source-meter":T11}
  T22 = typedef "cDLTS measurement Type Def.ctl" = cluster{"Name":string, "Comment":string, "Time":timestamp, "Folder":path, "DLTS properties":T16, "GUID":string}
  T23 = cluster{"Timestamps":ext[], "Temperatures":dbl[unit][]}
  T24 = cluster{"MFIA":bool, "Temperature controller":bool, "Source meter":bool}
  T25 = cluster{"Settings":T9, "DLTS properties":T16, "actual t_w":dbl[unit][], "R_peak":dbl[]}
  T26 = typedef "LVPointTypeDef.ctl" = cluster{"Horizontal":i16, "Vertical":i16}
  T27 = cluster{"Message":string, "C(t)":dbl[unit][], "t":dbl[unit][], "tau":dbl[unit][], "T":dbl[unit], "actual t_w":dbl[unit][], "R_peak":dbl[]}
  T28 = enum8{"Enabled", "Disabled", "Disabled and Grayed Out"}
  T29 = typedef "Semaphore RefNum" = refnum<k1>
  T30 = typedef "DialogType.ctl" = u16
  T31 = typedef "TaskbarProgressAPI.lvlib/Progress State.ctl" = i32
  T32 = cluster{"t":dbl[], "Capacitance transient":dbl[]}
  T33 = cluster{"Clipboard":bool, "dat":bool, "iso":bool, "Origin":bool, "Excel":bool}
  T34 = cluster{"T_s 50%":dbl[unit], "T_s 1-1/e":dbl[unit], "T_s 90%":dbl[unit], "T_s 95%":dbl[unit], "T_s 99%":dbl[unit]}
  T35 = enum16{"Canceled", "Clipboard", "Dat", "Iso", "Origin", "Excel"}
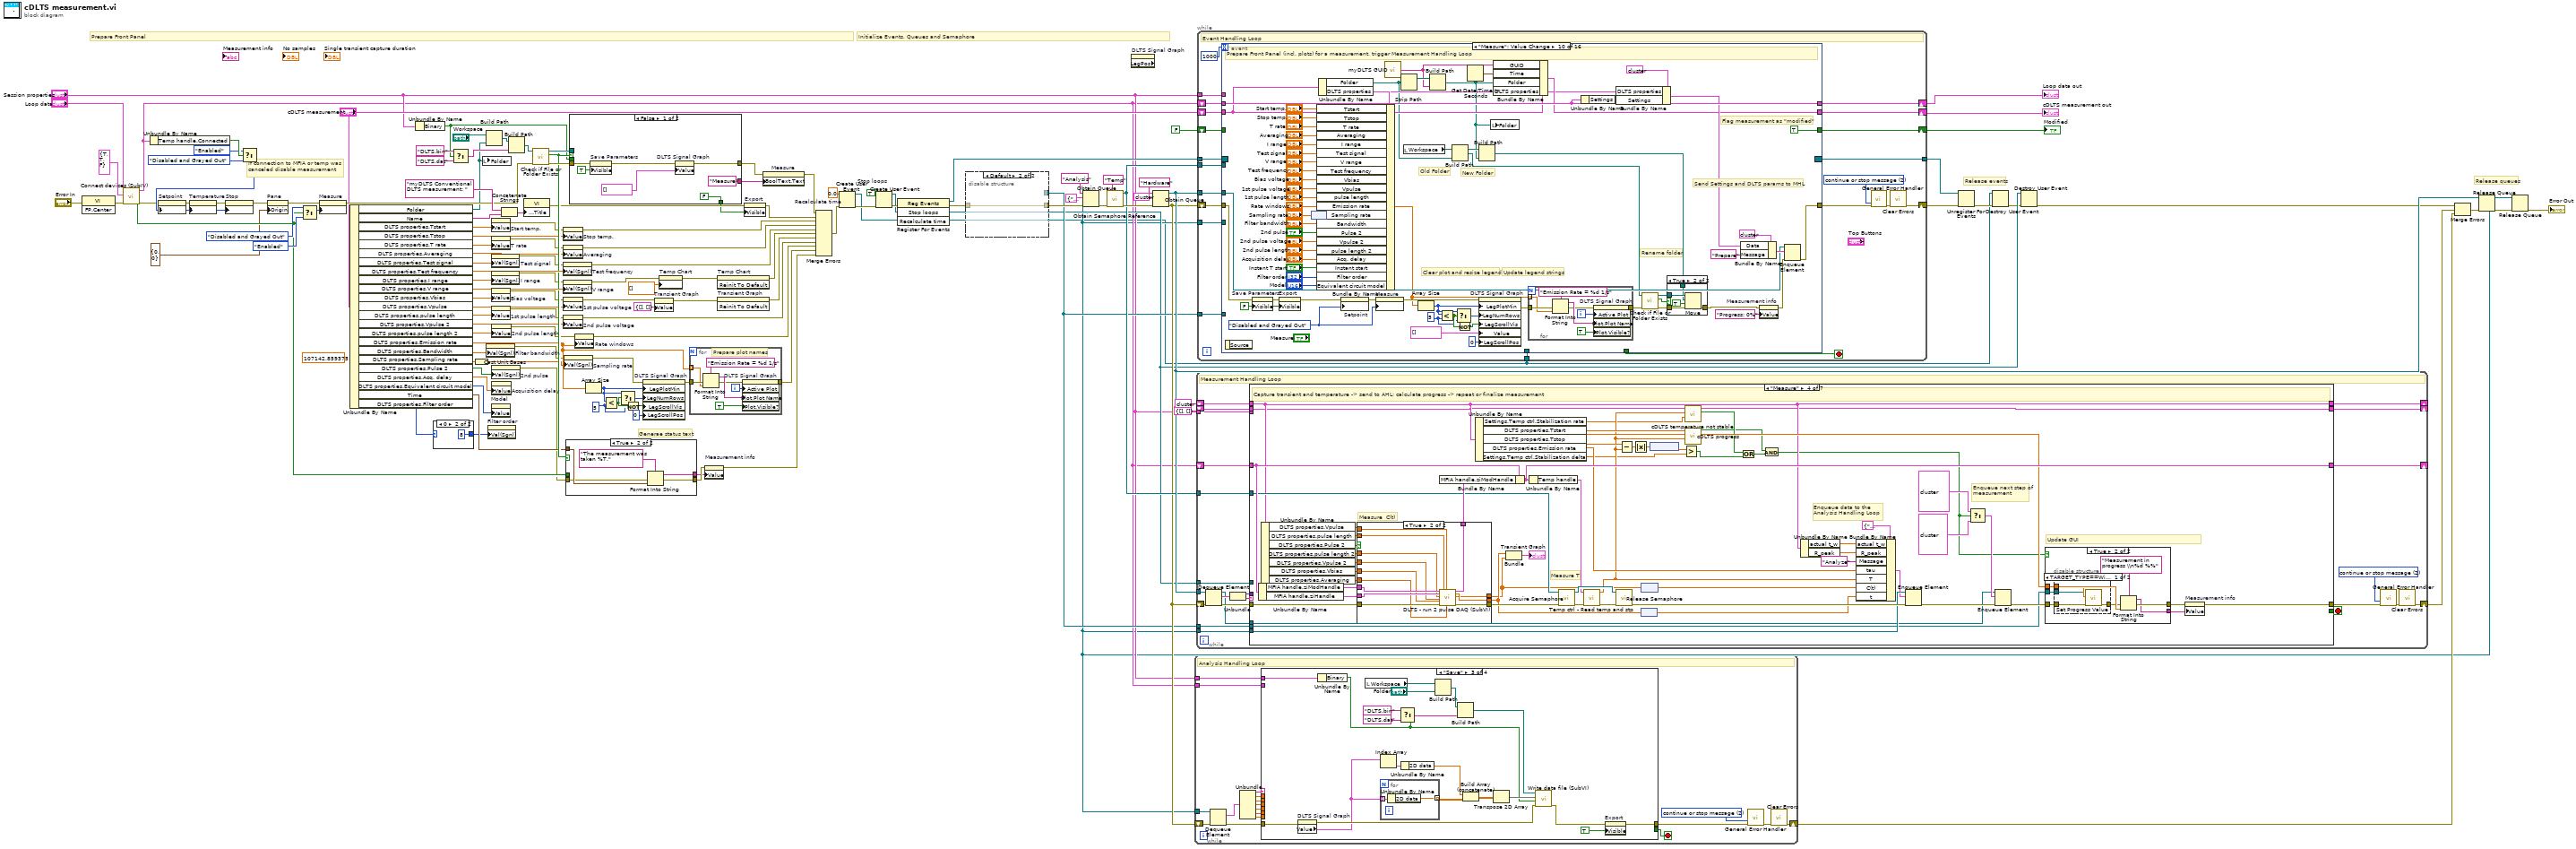
[diagram p0: block diagram]
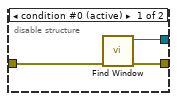
[diagram p2: hidden frame]
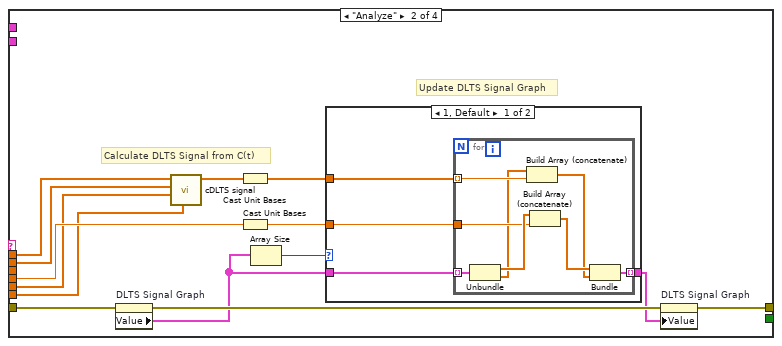
[diagram p5: hidden frame]
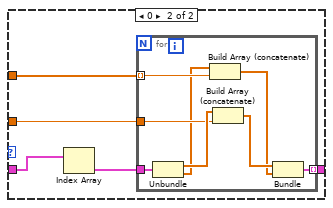
[diagram p6: hidden frame]
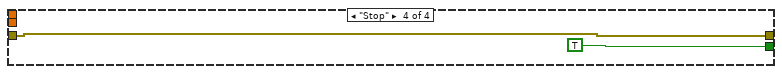
[diagram p7: hidden frame]
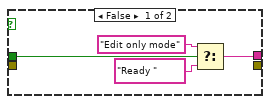
[diagram p8: hidden frame]
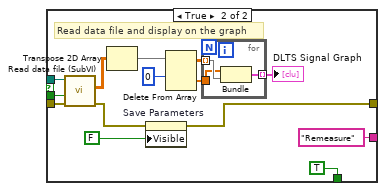
[diagram p9: hidden frame]
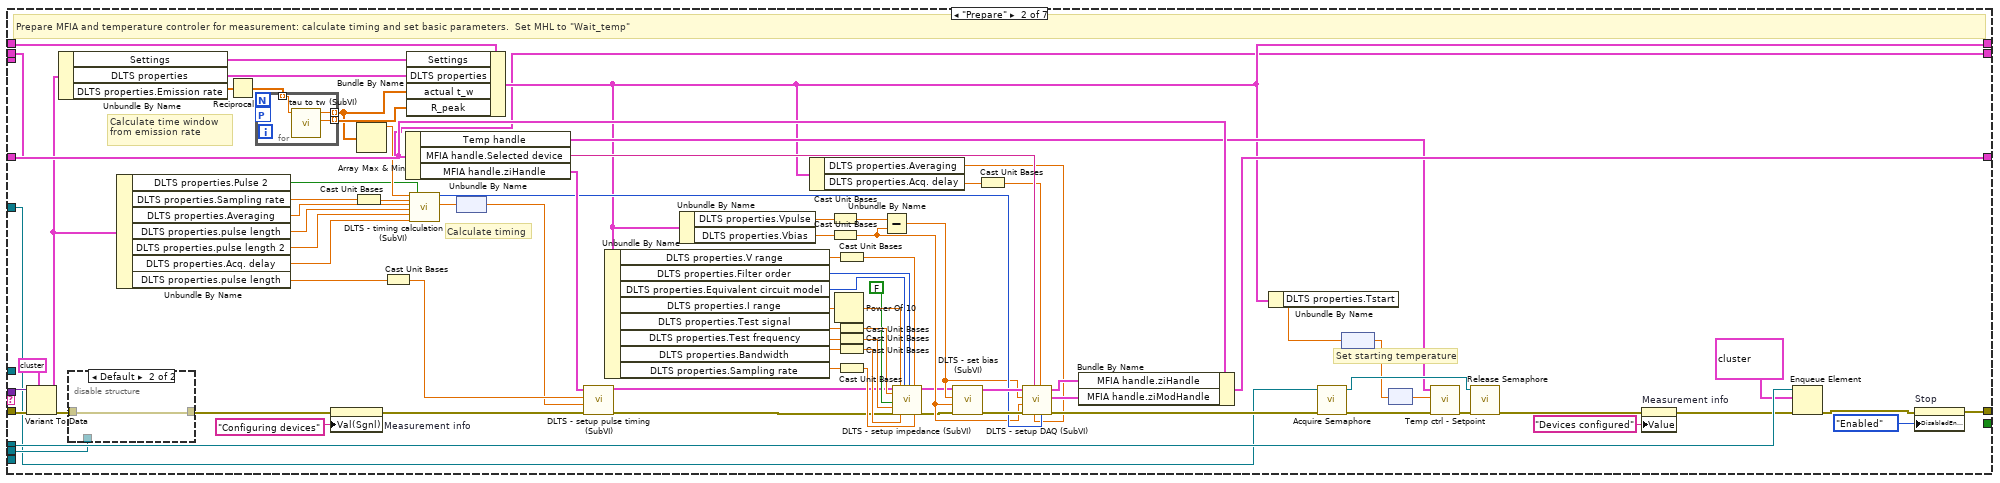
[diagram p11: hidden frame]
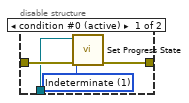
[diagram p12: hidden frame]
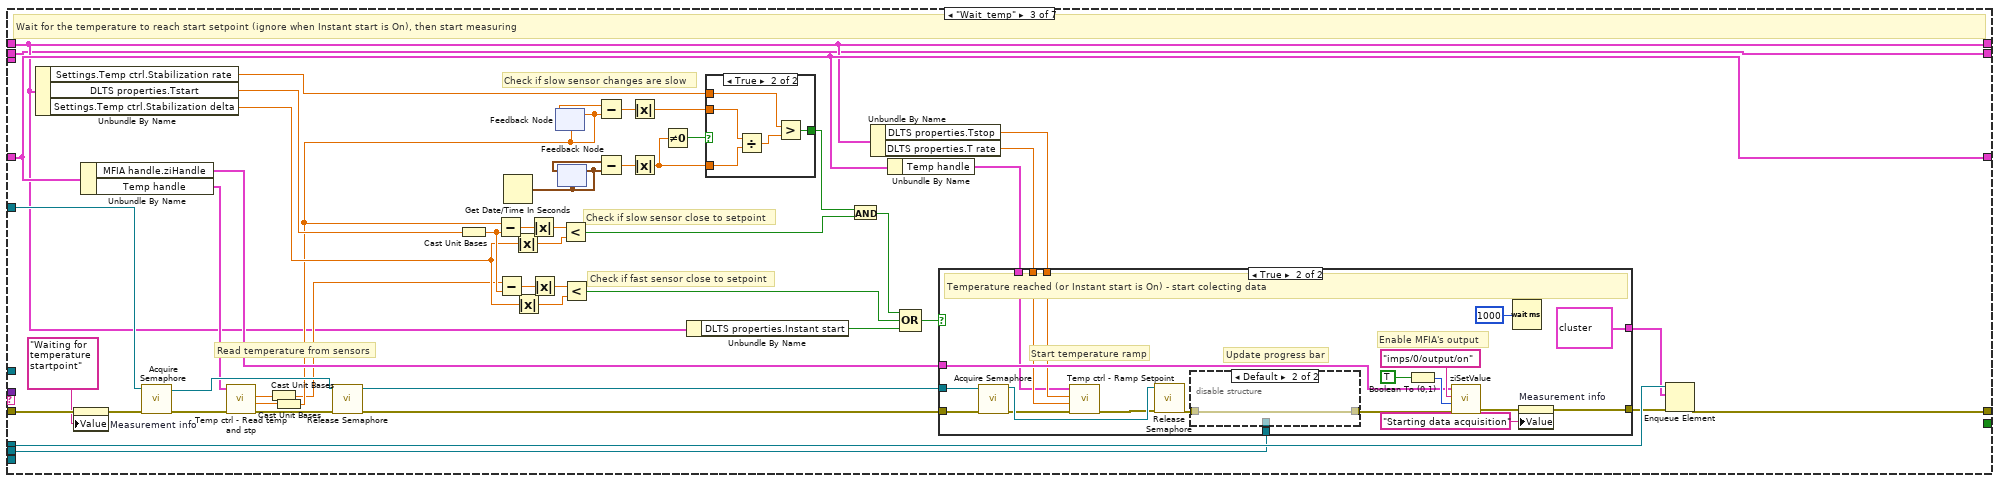
[diagram p13: hidden frame]
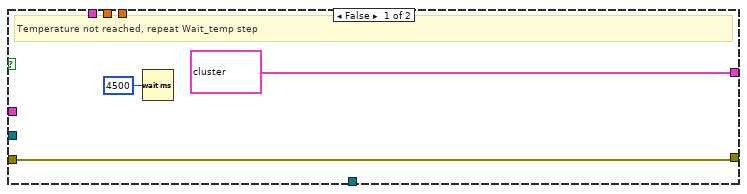
[diagram p14: hidden frame]
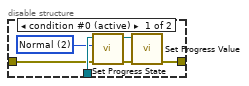
[diagram p15: hidden frame]
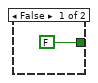
[diagram p16: hidden frame]
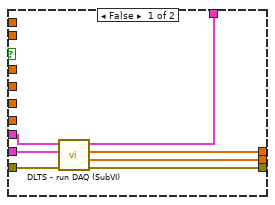
[diagram p17: hidden frame]
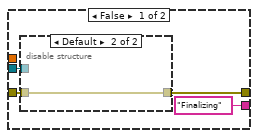
[diagram p18: hidden frame]
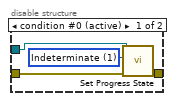
[diagram p19: hidden frame]
diagram:
  w17 = 0.0  # Recalculate time
  (unwired) dbl[unit] 107142.859375 ("Value (Signaling)")
  w51 = 5 ("y")
  w120 = TRUE  # Stop loops
  # "Release queues"
  # "Release events"
  # "Initialize Events, Queues and Semaphore"
  # "Generae status text"
  # "Prepare Front Panel"
  # "If connection to MFIA or temp was canceled disable measurement"
  n1 = invoke class="VI" method="FP.Center"(error in="Error In") -> (error out=w48:errorcluster)  [unwired: 2 in, 2 out]
  n2 = call "Connect devices (SubIV).vi"("Error In"=w48, "Devices"=T24 {"MFIA"=TRUE, "Temperature controller"=TRUE, "Source meter"=FALSE}, "Loop data in"="Loop data") -> ("Error Out"=w47:errorcluster, "Canceled"=w108:bool, "Loop data out"=w22:T3)  [unwired: 6 in]
  n3 = Unbundle By Name(w22) -> ("Temp handle.Connected"=w135:bool)
  n4 = Select(t=T28."Enabled" ("f"), s=w135, f=T28."Disabled and Grayed Out" ("Disabled")) -> (s? t:f=w91:T28)
  n5 = property on="Setpoint" class="DigNum (strict)"(error in=w47, "DisabledEnum"=w91) -> (error out=w136:errorcluster)  [unwired: 1 in, 1 out]
  n6 = property on="Temperature" class="DigNum (strict)"(error in=w136, "DisabledEnum"=w91) -> (error out=w18:errorcluster)  [unwired: 1 in, 1 out]
  n7 = property on="Stop" class="Bool"(error in=w18, "DisabledEnum"=w91) -> (error out=w49:errorcluster)  [unwired: 1 in, 1 out]
  n8 = property on="Pane" class="Pane"(error in=w49, "Origin"=T26 {"Horizontal"=0, "Vertical"=0}) -> (error out=w46:errorcluster)  [unwired: 1 in, 1 out]
  n9 = Select(t=T28."Disabled and Grayed Out" ("f"), s=w108, f=T28."Enabled") -> (s? t:f=w132:T28)
  n10 = property on="Measure" class="Bool"(error in=w46, "DisabledEnum"=w132) -> (error out=w101:errorcluster)  [unwired: 1 in, 1 out]
  n11 = Unbundle By Name("cDLTS measurement") -> ("Folder"=w12:path, "Name"=w103:string, "DLTS properties.Tstart"=w89:dbl[unit], "DLTS properties.Tstop"=w88:dbl[unit], "DLTS properties.T rate"=w87:dbl[unit], "DLTS properties.Averaging"=w85:dbl, "DLTS properties.Test signal"=w119:dbl[unit], "DLTS properties.Test frequency"=w118:dbl[unit], "DLTS properties.I range"=w117:dbl, "DLTS properties.V range"=w116:dbl[unit], "DLTS properties.Vbias"=w81:dbl[unit], "DLTS properties.Vpulse"=w79:dbl[unit], "DLTS properties.pulse length"=w78:dbl[unit], "DLTS properties.Vpulse 2"=w30:dbl[unit], "DLTS properties.pulse length 2"=w29:dbl[unit], "DLTS properties.Emission rate"=w45:dbl[unit][], "DLTS properties.Bandwidth"=w44:dbl[unit], "DLTS properties.Sampling rate"=w37:dbl[unit], "DLTS properties.Pulse 2"=w25:bool, "DLTS properties.Acq. delay"=w23:dbl[unit], "DLTS properties.Equivalent circuit model"=w8:u16, "Time"=w73:timestamp, "DLTS properties.Filter order"=w10:i32)
  n12 = Unbundle By Name("Session properties") -> ("Binary"=w35:bool)
  n13 = case shown="0" w10 {
    selector: w10 -> [w138 _]
    tunnel: [w138 8 ("Filter order")] -> w9
    frame Default {
    }
    frame 0 {
    }
  }
  n14 = Select(t="DLTS.bin", s=w35, f="DLTS.dat") -> (s? t:f=w114:string)
  n15 = Cast Unit Bases(0:w37) -> (2:w36:dbl)  [unwired: 1 in]
  n16 = local write "Folder"(w12) -> ()
  n17 = Build Path(base path="Workspace", name or relative path=w12) -> (appended path=w126:path)
  n18 = property on="Filter bandwidth" class="DigNum (strict)"("Val(Sgnl)"=w44) -> (error out=w38:errorcluster)  [unwired: 2 in, 1 out]
  n19 = property on="Filter order" class="DigNum (strict)"("Val(Sgnl)"=w9) -> ()  [unwired: 2 in, 2 out]
  n20 = property on="Start temp." class="DigNum (strict)"("Value"=w89) -> (error out=w86:errorcluster)  [unwired: 2 in, 1 out]
  n21 = property on="T rate" class="DigNum (strict)"("Value"=w87) -> (error out=w84:errorcluster)  [unwired: 2 in, 1 out]
  n22 = property on="Test signal" class="DigNum (strict)"("Val(Sgnl)"=w119) -> (error out=w82:errorcluster)  [unwired: 2 in, 1 out]
  n23 = property on="I range" class="Ring (strict)"("Val(Sgnl)"=w117) -> (error out=w83:errorcluster)  [unwired: 2 in, 1 out]
  n24 = property on="Bias voltage" class="DigNum (strict)"("Value"=w81) -> (error out=w80:errorcluster)  [unwired: 2 in, 1 out]
  n25 = property on="1st pulse length" class="DigNum (strict)"("Value"=w78) -> (error out=w28:errorcluster)  [unwired: 2 in, 1 out]
  n26 = property on="Model" class="Ring (strict)"("Value"=w8) -> ()  [unwired: 2 in, 2 out]
  n27 = property on="2nd pulse length" class="DigNum (strict)"("Value"=w29) -> (error out=w27:errorcluster)  [unwired: 2 in, 1 out]
  n28 = property on="2nd pulse" class="Bool (strict)"("Val(Sgnl)"=w25) -> (error out=w24:errorcluster)  [unwired: 2 in, 1 out]
  n29 = property on="Acquisition delay" class="DigNum (strict)"("Value"=w23) -> ()  [unwired: 2 in, 2 out]
  n30 = Concatenate Strings("myDLTS Conventional DLTS measurement: " ("string"), w103) -> (w104:string)
  n31 = Build Path(base path=w126, name or relative path=w114) -> (appended path=w125:path)
  n32 = property class="VI"("Front Panel.Title"=w104) -> (error out=w31:errorcluster)  [unwired: 2 in, 1 out]
  n33 = call <vilib>:"Check if File or Folder Exists.vi"("error in (no error)"=w101, "path"=w125) -> ("error out"=w123:errorcluster, "file or folder exists?"=w111:bool, "dup path"=w124:path)  [unwired: 7 in]
  n34 = property on="Stop temp." class="DigNum (strict)"(error in=w86, "Value"=w88) -> (error out=w77:errorcluster)  [unwired: 1 in, 1 out]
  n35 = property on="Averaging" class="DigNum (strict)"(error in=w84, "Value"=w85) -> (error out=w76:errorcluster)  [unwired: 1 in, 1 out]
  n36 = property on="Test frequency" class="DigNum (strict)"(error in=w82, "Val(Sgnl)"=w118) -> (error out=w75:errorcluster)  [unwired: 1 in, 1 out]
  n37 = property on="V range" class="Ring (strict)"(error in=w83, "Val(Sgnl)"=w116) -> (error out=w6:errorcluster)  [unwired: 1 in, 1 out]
  n38 = property on="1st pulse voltage" class="DigNum (strict)"(error in=w80, "Value"=w79) -> (error out=w4:errorcluster)  [unwired: 1 in, 1 out]
  n39 = property on="2nd pulse voltage" class="DigNum (strict)"(error in=w28, "Value"=w30) -> (error out=w26:errorcluster)  [unwired: 1 in, 1 out]
  n40 = property on="Sampling rate" class="Ring (strict)"(error in=w38, "Val(Sgnl)"=w36) -> (error out=w39:errorcluster)  [unwired: 1 in, 1 out]
  n41 = case shown="True" w111 {
    tunnel: w73 -> [_ w148]
    tunnel: [_ w147] -> w110
    tunnel: [w142 w146] -> w109
    tunnel: w108 -> [w143 _]
    tunnel: w24 -> [_ w144]
    frame False {
      n42 = Select(t="Edit only mode", s=w143, f="Ready ") -> (s? t:f=w142:string)
    }
    frame True {
      n43 = Format Into String(format string="The measurement was taken %T.", error in=w144, w148) -> (resulting string=w146:string, error out=w147:errorcluster)  [unwired: 1 in]
    }
  }
  n44 = case shown="False" w111 {
    tunnel: w35 -> [_ w169]
    tunnel: w124 -> [_ w168]
    tunnel: w123 -> [w154 w167]
    tunnel: [w151 w158] -> w98
    tunnel: ["Measure" ("Boolean Text.Text") "Remeasure" ("Boolean Text.Text")] -> w96
    tunnel: [FALSE ("Visible") TRUE ("Visible")] -> w21
    frame False {
      n45 = property on="Save Parameters" class="Bool (strict)"(error in=w154, "Visible"=TRUE) -> (error out=w150:errorcluster)  [unwired: 1 in, 1 out]
      n46 = property on="DLTS Signal Graph" class="XYGraph (strict)"(error in=w150, "Value"=cluster{"2D data":dbl[], "2D data":dbl[]}[] [] ("DLTS Signal Graph")) -> (error out=w151:errorcluster)  [unwired: 1 in, 1 out]
    }
    frame True {
      # "Read data file and display on the graph"
      n47 = call "Read data file (SubVI).vi"("error in"=w167, "Binary"=w169, "file path in"=w168) -> ("error out"=w165:errorcluster, "2D data"=w163:dbl[][])  [unwired: 5 in, 2 out]
      n48 = Transpose 2D Array(2D array=w163) -> (transposed array=w161:dbl[][])
      n49 = property on="Save Parameters" class="Bool (strict)"(error in=w165, "Visible"=FALSE) -> (error out=w158:errorcluster)  [unwired: 1 in, 1 out]
      n50 = Delete From Array(array=w161, index (row)=0 ("disabled index (col)")) -> (deleted portion=w159:dbl[], array with subset deleted=w160:dbl[][])  [unwired: 2 in]
      n51 = for {
        tunnel: w160 -> [w172] mode=indexing
        tunnel: w159 -> [w171]
        tunnel: [w170] -> w157 mode=indexing
        n52 = Bundle(w171, w172) -> (w170:cluster{dbl[], dbl[]})  [unwired: 1 in]
      }
      "DLTS Signal Graph" <- w157
    }
  }
  n53 = property on="Rate windows" class="Arr (strict)"(error in=w27, "Value"=w45) -> (error out=w74:errorcluster)  [unwired: 1 in, 1 out]
  n54 = Array Size(array=w45) -> (size(s)=w55:i32)
  n55 = Less?(x=w55, y=w51) -> (x < y?=w58:bool)
  n56 = Select(t=w55, s=w58, f=w51) -> (s? t:f=w56:i32)
  n57 = Not(x=w58) -> (.not. x?=w57:bool)
  n58 = property on="DLTS Signal Graph" class="XYGraph (strict)"(error in=w39, "LegPlotMin"=w55, "LegNumRows"=w56, "LegScrollVis"=w57, "LegScrollPos"=u32 0 ("Legend:Scroll Position")) -> (error out=w54:errorcluster)  [unwired: 1 in, 1 out]
  n59 = property on="Transient Graph" class="XYGraph (strict)"(error in=w4, "Value"=cluster{"t":dbl[], "Samples":dbl[]} {"t"=[], "Samples"=[]} ("Transient Graph")) -> (error out=w3:errorcluster)  [unwired: 1 in, 1 out]
  n60 = property on="Temp Chart" class="WFChart (strict)"(error in=w6, "History Data"=dbl[] []) -> (error out=w7:errorcluster)  [unwired: 1 in, 1 out]
  n61 = for {
    tunnel: w54 -> [w177]
    tunnel: w45 -> [w176] mode=indexing
    tunnel: [w175] -> w53
    i -> [w180]
    # "Prepare plot names"
    n62 = Format Into String(format string="Emission Rate = %d 1/s", error in=w177, w176) -> (resulting string=w179:string, error out=w178:errorcluster)  [unwired: 1 in]
    n63 = property on="DLTS Signal Graph" class="XYGraph (strict)"(error in=w178, "Active Plot"=w180, "Plot.Plot Name"=w179, "Plot.Visible?"=TRUE ("Plot.Visible")) -> (error out=w175:errorcluster)  [unwired: 1 in, 1 out]
  }
  n64 = property on="Measurement info" class="Str"(error in=w110, "Value"=w109) -> (error out=w72:errorcluster)  [unwired: 1 in, 1 out]
  n65 = invoke on="Temp Chart" class="WFChart (strict)" method="Reinit To Default"(error in=w7) -> (error out=w40:errorcluster)  [unwired: 2 in, 2 out]
  n66 = invoke on="Transient Graph" class="XYGraph (strict)" method="Reinit To Default"(error in=w3) -> (error out=w41:errorcluster)  [unwired: 2 in, 2 out]
  n67 = property on="Export" class="Bool"(error in=w31, "Visible"=w21) -> (error out=w32:errorcluster)  [unwired: 1 in, 1 out]
  n68 = property on="Measure" class="Bool"(error in=w98, "BoolText.Text"=w96) -> (error out=w97:errorcluster)  [unwired: 1 in, 1 out]
  n69 = Merge Errors(w97, w32, w77, w76, w75, w40, w41, w26, w74, w53, w72) -> (w15:errorcluster)
  n70 = Create User Event(user event datatype=w17, error in=w15) -> (user event=w11:refnum<user-event>, error out=w16:errorcluster)
  n71 = Create User Event(user event datatype=w120, error in=w16) -> (user event=w34:refnum<user-event>, error out=w121:errorcluster)
  n72 = register-events(error in=w121, w34, w11) -> (reference out=w122:refnum<event-registration>, error out=w61:errorcluster)  [unwired: 1 in]
  n73 = disable-structure shown="Default" {
    disable-tunnel: w61 -> [w183 w184]
    disable-tunnel: [w182 w184] -> w60
    disable-tunnel: [w181 _] -> w59
    frame condition #0 (active) {
      n74 = call <vilib>:"Find Window.vi"("error in (no error)"=w183) -> ("error out"=w182:errorcluster, "Window Handle"=w181:refnum<k24>)  [unwired: 9 in]
    }
    frame condition #1 {
    }
  }
  n75 = Obtain Queue(name (unnamed)="Analysis", element data type=T27 {"Message"="", "C(t)"=[], "t"=[], "tau"=[], "T"=0.0, "actual t_w"=[], "R_peak"=[]}, error in (no error)=w60) -> (queue out=w19:refnum<queue>, error out=w66:errorcluster)  [unwired: 2 in, 1 out]
  n76 = call <vilib>:"Obtain Semaphore Reference.vi"("error in (no error)"=w66, "name (unnamed)"="Temp") -> ("error out"=w71:errorcluster, "semaphore"=w69:T29)  [unwired: 3 in, 1 out]
  n77 = property on="DLTS Signal Graph" class="XYGraph (strict)" props=["LegPos"]() -> ()  [unwired: 2 in, 3 out]
  n78 = Obtain Queue(name (unnamed)="Hardware", element data type=cluster{"Data":variant, "Message":string} {"Data"=variant, "Message"=""}, error in (no error)=w71) -> (queue out=w105:refnum<queue>, error out=w65:errorcluster)  [unwired: 2 in, 1 out]
  n79 = while "Analysis Handling Loop" {
    shift-right: [w186] -> w62
    shift-left: w65 -> [w202]
    tunnel: w19 -> [w201]
    tunnel: "Session properties" -> [w187]
    tunnel: w22 -> [w185]
    stop <- w194 stop-if-true
    w191 = T30 2 items=["no dialog", "OK message", "continue or stop message", "OK message + warnings", "continue/stop + warnings"] ("type of dialog (OK msg:1)")
    # "Analysis Handling Loop"
    n80 = Dequeue Element(queue=w201, error in (no error)=w202) -> (element=w200:T27, error out=w199:errorcluster)  [unwired: 1 in, 2 out]
    n81 = Unbundle(w200) -> ("Message"=w196:string, "C(t)"=w197:dbl[unit][], "t"=w198:dbl[unit][], "tau"=w190:dbl[unit][], "T"=w195:dbl[unit], "actual t_w"=w189:dbl[unit][], "R_peak"=w188:dbl[])
    n82 = case shown="\"Save\"" w196 {
      tunnel: w199 -> [w203 w215 w262 w265]
      tunnel: w198 -> [_ w217 _ _]
      tunnel: w197 -> [_ w216 _ _]
      tunnel: [w203 w213 w245 w265] -> w193
      tunnel: w195 -> [_ w214 _ _]
      tunnel: [_ _ _ TRUE] -> w194
      tunnel: w190 -> [_ _ _ _]
      tunnel: w189 -> [_ w205 _ _]
      tunnel: w188 -> [_ w204 _ _]
      tunnel: w187 -> [_ _ w247 _]
      tunnel: w185 -> [_ _ _ _]
      frame "", Default {
      }
      frame "Analyze" {
        # "Calculate DLTS Signal from C(t)"
        # "Update DLTS Signal Graph"
        n83 = property on="DLTS Signal Graph" class="XYGraph (strict)"(error in=w215) -> (error out=w212:errorcluster, "Value"=w208:cluster{"2D data":dbl[], "2D data":dbl[]}[])  [unwired: 1 in, 1 out]
        n84 = call "cDLTS signal.vi"("R_peak"=w204, "t_w"=w205, "t"=w217, "C(t)"=w216) -> ("S"=w209:dbl[unit][])  [unwired: 5 in]
        n85 = Cast Unit Bases(0:w209) -> (2:w206:dbl[])  [unwired: 1 in]
        n86 = Cast Unit Bases(0:w214) -> (2:w210:dbl)  [unwired: 1 in]
        n87 = Array Size(array=w208) -> (size(s)=w207:i32)
        n88 = case shown="1, Default" w207 {
          tunnel: w208 -> [w221 w231]
          tunnel: [w220 w234] -> w211
          tunnel: w210 -> [w219 w233]
          tunnel: w206 -> [w218 w232]
          frame 1, Default {
            n89 = for {
              tunnel: w221 -> [w229] mode=indexing
              tunnel: w219 -> [w226]
              tunnel: [w228] -> w220 mode=indexing
              tunnel: w218 -> [w224] mode=indexing
              n90 = Unbundle(w229) -> ("2D data"=w227:dbl[], "2D data"=w223:dbl[])
              n91 = Build Array (concatenate)(w223, w224) -> (w222:dbl[])
              n92 = Build Array (concatenate)(w227, w226) -> (w225:dbl[])
              n93 = Bundle(w225, w222) -> (w228:cluster{dbl[], dbl[]})  [unwired: 1 in]
            }
          }
          frame 0 {
            n94 = Index Array(array=w231) -> (element=w230:cluster{"2D data":dbl[], "2D data":dbl[]})  [unwired: 1 in]
            n95 = for {
              tunnel: w230 -> [w242]
              tunnel: w233 -> [w239]
              tunnel: [w241] -> w234 mode=indexing
              tunnel: w232 -> [w237] mode=indexing
              n96 = Unbundle(w242) -> ("2D data"=w240:dbl[], "2D data"=w236:dbl[])
              n97 = Build Array (concatenate)(w236, w237) -> (w235:dbl[])
              n98 = Build Array (concatenate)(w240, w239) -> (w238:dbl[])
              n99 = Bundle(w238, w235) -> (w241:cluster{dbl[], dbl[]})  [unwired: 1 in]
            }
          }
        }
        n100 = property on="DLTS Signal Graph" class="XYGraph (strict)"(error in=w212, "Value"=w211) -> (error out=w213:errorcluster)  [unwired: 1 in, 1 out]
      }
      frame "Save" {
        n101 = property on="DLTS Signal Graph" class="XYGraph (strict)"(error in=w262) -> (error out=w255:errorcluster, "Value"=w251:cluster{"2D data":dbl[], "2D data":dbl[]}[])  [unwired: 1 in, 1 out]
        n102 = Unbundle By Name(w247) -> ("Binary"=w246:bool)
        n103 = local read "Workspace"() -> (w259:path)
        n104 = Index Array(array=w251) -> (element=w250:cluster{"2D data":dbl[], "2D data":dbl[]})  [unwired: 1 in]
        n105 = for {
          tunnel: [w263] -> w253 mode=indexing
          tunnel: w251 -> [w264] mode=indexing
          n106 = Unbundle By Name(w264) -> ("2D data"=w263:dbl[])
        }
        n107 = Select(t="DLTS.bin", s=w246, f="DLTS.dat") -> (s? t:f=w260:string)
        n108 = Unbundle By Name(w250) -> ("2D data"=w249:dbl[])
        n109 = Build Path(base path=w259, name or relative path="Folder") -> (appended path=w261:path)
        n110 = Build Path(base path=w261, name or relative path=w260) -> (appended path=w258:path)
        n111 = Build Array (concatenate)(w249, w253) -> (w252:dbl[][])
        n112 = Transpose 2D Array(2D array=w252) -> (transposed array=w254:dbl[][])
        n113 = call "Write data file (SubVI).vi"("error in"=w255, "Binary"=w246, "2D data"=w254, "file path in"=w258) -> ("error out"=w248:errorcluster)  [unwired: 6 in, 1 out]
        n114 = property on="Export" class="Bool"(error in=w248, "Visible"=TRUE) -> (error out=w245:errorcluster)  [unwired: 1 in, 1 out]
      }
      frame "Stop" {
      }
    }
    n115 = call <vilib>:"General Error Handler.vi"("type of dialog (OK msg:1)"=w191, "error in (no error)"=w193) -> ("error out"=w192:errorcluster)  [unwired: 9 in, 4 out]
    n116 = call <vilib>:"Clear Errors.vi"("error in (no error)"=w192) -> ("error out"=w186:errorcluster)  [unwired: 5 in, 1 out]
  }
  n117 = while "Measurement Handling Loop" {
    tunnel: w105 -> [w279]
    shift-right: [w269] -> w92
    shift-left: w65 -> [w289]
    tunnel: w34 -> [w284]
    tunnel: w69 -> [w281]
    shift-right: [w280] -> _
    shift-left: T25 {"Settings"={"MFIA"={"Address"="", "Use compensation"=FALSE, "Shut down gracefully"=FALSE}, "Temp ctrl"={"Gain (P)"=0.0, "Reset (I)"=0.0, "Rate (D)"=0.0, "Stabilization rate"=0.0, "Stabilization delta"=0.0, "Type"=enum."Custom", "Custom temp ctrl"={"VISA resource name"=""}, "Lakeshore 325"={"VISA name"="", "Loop"=0, "Heater Range"=0, "Heater Resistance"=0, "Sample sensor"=0, "Fast sensor"=0, "Slow sensor"=0}, "Lakeshore 331"={"VISA name"="", "Loop"=1, "Heater Range"=0, "Sample sensor"=0, "Fast sensor"=0, "Slow sensor"=0}, "Lakeshore 332"={"VISA name"="", "Loop"=1, "Heater Range"=0, "Sample sensor"=0, "Fast sensor"=0, "Slow sensor"=0}, "Lakeshore 335"={"VISA name"="", "Loop"=1, "Sample sensor"=0, "Fast sensor"=0, "Slow sensor"=0, "Heater Range"=0, "Output mode"=enum."Off"}, "Lakeshore 336"={"VISA name"="", "Loop"=1, "Output mode"=enum."Off", "Max current"=1.0, "Heater resistance"=1, "Sample sensor"=1, "Slow sensor"=1, "Fast sensor"=1}}, "Source-meter"={"Type"=enum."Custom", "Custom source-meter"={"VISA resource name"=""}, "Keithley 2600"={"VISA name"="", "Ignore ID Query"=FALSE, "SMU"=enum."Channel A"}, "Keithley 2400 Series"={"VISA name"="", "Ignore ID Query"=FALSE}}, "Other"={"Enable OriginLab"=FALSE, "Reader mode"=FALSE, "Auto-save"=FALSE}, "Defaults"={"IV properties"={"T"=0.0, "Vstart"=0.0, "Vstop"=0.0, "Vpoints"=0.0, "Settling"=0.01, "I limit"=0.1, "Log mapping"=FALSE, "Averaging"=0.0}, "CV properties"={"T"=0.0, "Vstart"=0.0, "Vstop"=0.0, "Vpoints"=0.0, "Precision"=enum."Low (Fast)", "Test signal"=0.0, "Auto I range"=FALSE, "Test frequency"=0.0, "I range"=0.0, "V range"=0.0, "Log mapping"=FALSE, "Rel perm"=0.0, "Area"=0.0, "Equivalent circuit model"=0}, "DLTS properties"={"Tstart"=0.0, "Instant start"=FALSE, "Tstop"=0.0, "T rate"=0.0, "Test signal"=0.0, "Test frequency"=0.0, "Bandwidth"=0.0, "Averaging"=0.0, "Vbias"=0.0, "Vpulse"=0.0, "pulse length"=0.0, "Pulse 2"=FALSE, "Vpulse 2"=0.0, "pulse length 2"=0.0, "I range"=0.0, "V range"=0.0, "Emission rate"=[], "Sampling rate"=0.0, "Acq. delay"=0.0, "Filter order"=0, "Equivalent circuit model"=0}, "LDLTS properties"={"T"=0.0, "Test signal"=0.0, "Test frequency"=0.0, "Bandwidth"=0.0, "Averaging"=0.0, "Vbias"=0.0, "Vpulse"=0.0, "pulse length"=0.0, "Pulse 2"=FALSE, "Vpulse 2"=0.0, "pulse length 2"=0.0, "I range"=-2.0, "V range"=10.0, "Sampling rate"=0.0, "Acq. delay"=0.0, "Sampling time"=0.0, "Filter order"=0, "Equivalent circuit model"=0}}}, "DLTS properties"={"Tstart"=0.0, "Instant start"=FALSE, "Tstop"=0.0, "T rate"=0.0, "Test signal"=0.0, "Test frequency"=0.0, "Bandwidth"=0.0, "Averaging"=0.0, "Vbias"=0.0, "Vpulse"=0.0, "pulse length"=0.0, "Pulse 2"=FALSE, "Vpulse 2"=0.0, "pulse length 2"=0.0, "I range"=0.0, "V range"=0.0, "Emission rate"=[], "Sampling rate"=0.0, "Acq. delay"=0.0, "Filter order"=0, "Equivalent circuit model"=0}, "actual t_w"=[], "R_peak"=[]} -> [w278]
    shift-right: [w277] -> _
    shift-left: w22 -> [w282]
    tunnel: w19 -> [w275]
    tunnel: w59 -> [w274]
    tunnel: "Session properties" -> [w270]
    shift-right: [w268] -> _
    shift-left: T23 {"Timestamps"=[], "Temperatures"=[]} ("Temperature history out") -> [w267]
    stop <- w283 stop-if-true
    w271 = T30 2 items=["no dialog", "OK message", "continue or stop message", "OK message + warnings", "continue/stop + warnings"] ("type of dialog (OK msg:1)")
    # "Measurement Handling Loop"
    n118 = Dequeue Element(queue=w279, error in (no error)=w289) -> (queue out=w276:refnum<queue>, element=w288:cluster{"Data":variant, "Message":string}, error out=w285:errorcluster)  [unwired: 1 in, 1 out]
    n119 = Unbundle(w288) -> ("Data"=w286:variant, "Message"=w287:string)
    n120 = case shown="\"Measure\"" w287 {
      tunnel: w286 -> [_ w375 _ _ _ _ _]
      tunnel: w285 -> [w293 w376 w409 w529 w606 w617 w661]
      tunnel: w284 -> [_ _ _ _ _ _ w660]
      tunnel: [w293 w373 w404 w511 w586 w627 w654] -> w272
      tunnel: [_ _ _ _ _ _ TRUE] -> w283
      tunnel: w282 -> [w291 w360 w402 w526 w594 w630 w656]
      tunnel: w281 -> [_ w341 w434 w522 w602 _ _]
      tunnel: [w292 w301 w386 w498 w601 w629 w657] -> w280
      tunnel: w276 -> [_ w364 w412 w512 _ w628 _]
      tunnel: w278 -> [w292 w352 w386 w498 w601 w629 w657]
      tunnel: [w291 w356 w402 w523 w593 w630 w656] -> w277
      tunnel: w275 -> [_ _ _ w520 w605 _ w653]
      tunnel: w274 -> [_ w353 w403 w505 w607 w615 _]
      tunnel: w270 -> [_ _ _ _ _ _ _]
      tunnel: [w290 w294 w385 w484 w571 w614 w651] -> w268
      tunnel: w267 -> [w290 w294 w385 w483 w571 w614 w651]
      frame "", Default {
      }
      frame "Prepare" {
        # "Set starting temperature"
        # "Calculate timing"
        # "Calculate time window from emission rate"
        # "Prepare MFIA and temperature controler for measurement: calculate timing and set basic parameters.  Set MHL to \"Wait_temp\""
        n121 = Variant To Data(error in=w376, type=cluster{"Settings":T9, "DLTS properties":T16} {"Settings"={"MFIA"={"Address"="", "Use compensation"=TRUE, "Shut down gracefully"=FALSE}, "Temp ctrl"={"Gain (P)"=0.0, "Reset (I)"=0.0, "Rate (D)"=0.0, "Stabilization rate"=0.0, "Stabilization delta"=0.0, "Type"=enum."Lake Shore 325", "Custom temp ctrl"={"VISA resource name"=""}, "Lakeshore 325"={"VISA name"="", "Loop"=0, "Heater Range"=1, "Heater Resistance"=0, "Sample sensor"=0, "Fast sensor"=0, "Slow sensor"=0}, "Lakeshore 331"={"VISA name"="", "Loop"=1, "Heater Range"=0, "Sample sensor"=0, "Fast sensor"=0, "Slow sensor"=0}, "Lakeshore 332"={"VISA name"="", "Loop"=1, "Heater Range"=0, "Sample sensor"=0, "Fast sensor"=0, "Slow sensor"=0}, "Lakeshore 335"={"VISA name"="", "Loop"=1, "Sample sensor"=0, "Fast sensor"=0, "Slow sensor"=0, "Heater Range"=0, "Output mode"=enum."Off"}, "Lakeshore 336"={"VISA name"="", "Loop"=1, "Output mode"=enum."Off", "Max current"=1.0, "Heater resistance"=1, "Sample sensor"=1, "Slow sensor"=1, "Fast sensor"=1}}, "Source-meter"={"Type"=enum."Custom", "Custom source-meter"={"VISA resource name"=""}, "Keithley 2600"={"VISA name"="", "Ignore ID Query"=FALSE, "SMU"=enum."Channel A"}, "Keithley 2400 Series"={"VISA name"="", "Ignore ID Query"=FALSE}}, "Other"={"Enable OriginLab"=FALSE, "Reader mode"=FALSE, "Auto-save"=FALSE}, "Defaults"={"IV properties"={"T"=0.0, "Vstart"=-0.5, "Vstop"=0.5, "Vpoints"=10.0, "Settling"=0.01, "I limit"=0.1, "Log mapping"=FALSE, "Averaging"=0.0}, "CV properties"={"T"=0.0, "Vstart"=-0.5, "Vstop"=0.5, "Vpoints"=10.0, "Precision"=enum."Normal", "Test signal"=0.01, "Auto I range"=FALSE, "Test frequency"=100000.0, "I range"=-2.0, "V range"=10.0, "Log mapping"=FALSE, "Rel perm"=0.0, "Area"=0.0, "Equivalent circuit model"=0}, "DLTS properties"={"Tstart"=0.0, "Instant start"=FALSE, "Tstop"=0.0, "T rate"=0.0, "Test signal"=0.0, "Test frequency"=0.0, "Bandwidth"=0.0, "Averaging"=0.0, "Vbias"=0.0, "Vpulse"=0.0, "pulse length"=0.0, "Pulse 2"=FALSE, "Vpulse 2"=0.0, "pulse length 2"=0.0, "I range"=-2.0, "V range"=10.0, "Emission rate"=[], "Sampling rate"=0.0, "Acq. delay"=0.0, "Filter order"=0, "Equivalent circuit model"=0}, "LDLTS properties"={"T"=0.0, "Test signal"=0.0, "Test frequency"=0.0, "Bandwidth"=0.0, "Averaging"=0.0, "Vbias"=0.0, "Vpulse"=0.0, "pulse length"=0.0, "Pulse 2"=FALSE, "Vpulse 2"=0.0, "pulse length 2"=0.0, "I range"=-2.0, "V range"=10.0, "Sampling rate"=0.0, "Acq. delay"=0.0, "Sampling time"=0.0, "Filter order"=0, "Equivalent circuit model"=0}}}, "DLTS properties"={"Tstart"=0.0, "Instant start"=FALSE, "Tstop"=0.0, "T rate"=0.0, "Test signal"=0.0, "Test frequency"=0.0, "Bandwidth"=0.0, "Averaging"=0.0, "Vbias"=0.0, "Vpulse"=0.0, "pulse length"=0.0, "Pulse 2"=FALSE, "Vpulse 2"=0.0, "pulse length 2"=0.0, "I range"=-2.0, "V range"=10.0, "Emission rate"=[], "Sampling rate"=0.0, "Acq. delay"=0.0, "Filter order"=0, "Equivalent circuit model"=0}}, Variant=w375) -> (data=w349:cluster{"Settings":T9, "DLTS properties":T16}, error out=w355:errorcluster)
        n122 = Unbundle By Name(w349) -> ("Settings"=w351:T9, "DLTS properties"=w350:T16, "DLTS properties.Emission rate"=w348:dbl[unit][])
        n123 = disable-structure shown="Default" {
          disable-tunnel: w355 -> [w380 w381]
          disable-tunnel: [w379 w381] -> w354
          disable-tunnel: w353 -> [w378 _]
          frame condition #0 (active) {
            w377 = T31 1 items=["NoProgress"=0, "Indeterminate"=1, "Normal"=2, "Error"=4, "Paused"=8] ("State (No Progress)")
            n124 = call <vilib>:"Set Progress State.vi"("error in (no error)"=w380, "State (No Progress)"=w377, "Window Handle"=w378) -> ("error out"=w379:errorcluster)  [unwired: 7 in, 1 out]
          }
          frame condition #1 {
          }
        }
        n125 = Unbundle By Name(w349) -> ("DLTS properties.Pulse 2"=w329:bool, "DLTS properties.Sampling rate"=w317:dbl[unit], "DLTS properties.Averaging"=w320:dbl, "DLTS properties.pulse length"=w319:dbl[unit], "DLTS properties.pulse length 2"=w318:dbl[unit], "DLTS properties.Acq. delay"=w316:dbl[unit], "DLTS properties.pulse length"=w315:dbl[unit])
        n126 = Reciprocal(x=w348) -> (1/x=w347:dbl[unit][])
        n127 = for {
          tunnel: w347 -> [w384] mode=indexing
          tunnel: [w383] -> w345 mode=indexing
          tunnel: [w382] -> w346 mode=indexing
          workers-P: _ -> [_]
          n128 = call "tau to tw (SubVI).vi"("tau"=w384) -> ("R(t_w)"=w382:dbl, "t_w"=w383:dbl[unit])  [unwired: 9 in]
        }
        n129 = property on="Measurement info" class="Str"(error in=w354, "Val(Sgnl)"="Configuring devices" ("Value (Signaling)")) -> (error out=w366:errorcluster)  [unwired: 1 in, 1 out]
        n130 = Cast Unit Bases(0:w317) -> (2:w332:dbl)  [unwired: 1 in]
        n131 = Array Max & Min(array=w345) -> (max value=w333:dbl[unit])  [unwired: 3 out]
        n132 = Cast Unit Bases(0:w315) -> (2:w368:dbl)  [unwired: 1 in]
        n133 = Unbundle By Name(w360) -> ("Temp handle"=w339:T5, "MFIA handle.Selected device"=w369:string, "MFIA handle.ziHandle"=w371:T19)
        n134 = Bundle By Name(cluster=w352, "Settings"=w351, "DLTS properties"=w350, "actual t_w"=w345, "R_peak"=w346) -> (w301:T25)
        n135 = call-poly "DLTS - timing calculation (SubVI).vi"("Time window"=w333, "Sampling rate"=w332, "Averaging"=w320, "1st pulse duration"=w319, "2nd pulse duration"=w318, "Acquisition delay"=w316, "2 pulse mode"=w329) -> ("Number of samples"=w336:i32, "Pulse off time"=w335:dbl[unit])  [unwired: 10 in, 1 out]
        n136 = node(w335) -> (w334:dbl)
        n137 = call "DLTS - setup pulse timing (SubVI).vi"("error in (no error)"=w366, "TUpulse off time"=w334, "TUpulse on time"=w368, "Handle Out in"=w371) -> ("error out"=w300:errorcluster, "Handle Out out"=w299:T19)  [unwired: 6 in]
        n138 = Unbundle By Name(w301) -> ("DLTS properties.V range"=w307:dbl[unit], "DLTS properties.Filter order"=w296:i32, "DLTS properties.Equivalent circuit model"=w295:u16, "DLTS properties.I range"=w308:dbl, "DLTS properties.Test signal"=w306:dbl[unit], "DLTS properties.Test frequency"=w305:dbl[unit], "DLTS properties.Bandwidth"=w304:dbl[unit], "DLTS properties.Sampling rate"=w303:dbl[unit])
        n139 = Unbundle By Name(w301) -> ("DLTS properties.Vpulse"=w323:dbl[unit], "DLTS properties.Vbias"=w324:dbl[unit])
        n140 = Unbundle By Name(w301) -> ("DLTS properties.Averaging"=w326:dbl, "DLTS properties.Acq. delay"=w328:dbl[unit])
        n141 = Cast Unit Bases(0:w323) -> (2:w325:dbl)  [unwired: 1 in]
        n142 = Cast Unit Bases(0:w324) -> (2:w321:dbl)  [unwired: 1 in]
        n143 = Power Of 10(x=w308) -> (10^x=w310:dbl)
        n144 = Cast Unit Bases(0:w307) -> (2:w309:dbl)  [unwired: 1 in]
        n145 = Cast Unit Bases(0:w306) -> (2:w311:dbl)  [unwired: 1 in]
        n146 = Cast Unit Bases(0:w305) -> (2:w312:dbl)  [unwired: 1 in]
        n147 = Cast Unit Bases(0:w304) -> (2:w313:dbl)  [unwired: 1 in]
        n148 = Cast Unit Bases(0:w303) -> (2:w314:dbl)  [unwired: 1 in]
        n149 = Subtract(x=w325, y=w321) -> (x-y=w322:dbl)
        n150 = call "DLTS - setup impedance (SubVI).vi"("Handle Out in"=w299, "IMPS test signal"=w311, "Output on"=FALSE, "IMPS test freq"=w312, "error in (no error)"=w300, "IMPS current range"=w310, "IMPS  bandwidth"=w313, "Equivalent circuit model"=w295, "Filter order"=w296, "IMPS output range"=w309, "IMPS demod sampling rate"=w314) -> ("Handle Out out"=w298:T19, "error out"=w297:errorcluster)  [unwired: 7 in]
        n151 = call "DLTS - set bias (SubVI).vi"("error in (no error)"=w297, "AUX offset"=w321, "AUX scale"=w322, "ziHandle"=w298) -> ("error out"=w370:errorcluster, "Handle Out"=w359:T19)  [unwired: 6 in]
        n152 = Cast Unit Bases(0:w328) -> (2:w327:dbl)  [unwired: 1 in]
        n153 = call "DLTS - setup DAQ (SubVI).vi"("No. samples"=w336, "post trigger delay"=w327, "No. repetitions (avg)"=w326, "Selected device"=w369, "error in (no error)"=w370, "AUX offset"=w321, "AUX scale"=w322, "Handle in"=w359) -> ("error out"=w344:errorcluster, "ModHandle Out"=w358:T20, "Handle Out"=w357:T19)  [unwired: 1 in]
        n154 = Bundle By Name(cluster=w360, "MFIA handle.ziHandle"=w357, "MFIA handle.ziModHandle"=w358) -> (w356:T3)
        n155 = Unbundle By Name(w301) -> ("DLTS properties.Tstart"=w331:dbl[unit])
        n156 = call <vilib>:"Acquire Semaphore.vi"("error in (no error)"=w344, "semaphore"=w341) -> ("error out"=w338:errorcluster, "semaphore out"=w342:T29)  [unwired: 3 in, 1 out]
        n157 = node(w331) -> (w330:dbl)
        n158 = node(w330) -> (w340:dbl[unit])
        n159 = call "Temp ctrl - Setpoint.vi"("Error In"=w338, "Setpoint"=w340, "Temp handle"=w339) -> ("Error Out"=w337:errorcluster)  [unwired: 8 in]
        n160 = call <vilib>:"Release Semaphore.vi"("error in (no error)"=w337, "semaphore"=w342) -> ("error out"=w343:errorcluster)  [unwired: 4 in, 1 out]
        n161 = property on="Measurement info" class="Str"(error in=w343, "Value"="Devices configured" ("Measurement info")) -> (error out=w363:errorcluster)  [unwired: 1 in, 1 out]
        n162 = Enqueue Element(queue=w364, element=cluster{"Data":variant, "Message":string} {"Data"=variant, "Message"="Wait_temp"}, error in (no error)=w363) -> (error out=w362:errorcluster)  [unwired: 1 in, 2 out]
        n163 = property on="Stop" class="Bool"(error in=w362, "DisabledEnum"=T28."Enabled" ("Disabled")) -> (error out=w373:errorcluster)  [unwired: 1 in, 1 out]
      }
      frame "Wait_temp" {
        # "Read temperature from sensors"
        # "Check if fast sensor close to setpoint"
        # "Check if slow sensor changes are slow"
        # "Check if slow sensor close to setpoint"
        # "Wait for the temperature to reach start setpoint (ignore when Instant start is On), then start measuring"
        n164 = Unbundle By Name(w386) -> ("Settings.Temp ctrl.Stabilization rate"=w418:dbl, "DLTS properties.Tstart"=w419:dbl[unit], "Settings.Temp ctrl.Stabilization delta"=w413:dbl)
        n165 = property on="Measurement info" class="Str"(error in=w409, "Value"="Waiting for temperature startpoint" ("Measurement info")) -> (error out=w410:errorcluster)  [unwired: 1 in, 1 out]
        n166 = Unbundle By Name(w402) -> ("MFIA handle.ziHandle"=w405:T19, "Temp handle"=w399:T5)
        n167 = call <vilib>:"Acquire Semaphore.vi"("error in (no error)"=w410, "semaphore"=w434) -> ("error out"=w398:errorcluster, "semaphore out"=w433:T29)  [unwired: 3 in, 1 out]
        n168 = call "Temp ctrl - Read temp and stp.vi"("Error In"=w398, "Temp handle"=w399) -> ("Error Out"=w397:errorcluster, "Slow changing temp"=w388:dbl[unit], "Fast changing temp"=w387:dbl[unit])  [unwired: 2 in, 2 out]
        n169 = Cast Unit Bases(0:w387) -> (2:w395:dbl)  [unwired: 1 in]
        n170 = Cast Unit Bases(0:w388) -> (2:w396:dbl)  [unwired: 1 in]
        n171 = call <vilib>:"Release Semaphore.vi"("error in (no error)"=w397, "semaphore"=w433) -> ("error out"=w406:errorcluster, "semaphore out"=w400:T29)  [unwired: 4 in]
        n172 = Cast Unit Bases(0:w419) -> (2:w414:dbl)  [unwired: 1 in]
        n173 = Subtract(x=w396, y=w414) -> (x-y=w427:dbl)
        n174 = Subtract(x=w395, y=w414) -> (x-y=w417:dbl)
        n175 = Get Date/Time In Seconds() -> (seconds since 1Jan1904=w420:timestamp)
        n176 = Absolute Value(x=w413) -> (abs(x)=w425:dbl)
        n177 = Absolute Value(x=w413) -> (abs(x)=w415:dbl)
        n178 = Absolute Value(x=w427) -> (abs(x)=w426:dbl)
        n179 = Absolute Value(x=w417) -> (abs(x)=w416:dbl)
        n180 = feedback #1(w396) -> (w421:dbl)
        n181 = feedback-in #1(w396) -> ()
        n182 = feedback-in #2(w420) -> ()
        n183 = feedback #2(w420) -> (w422:timestamp)
        n184 = Less?(x=w426, y=w425) -> (x < y?=w423:bool)
        n185 = Less?(x=w416, y=w415) -> (x < y?=w391:bool)
        n186 = Subtract(x=w421, y=w396) -> (x-y=w432:dbl)
        n187 = Subtract(x=w422, y=w420) -> (x-y=w431:dbl)
        n188 = Absolute Value(x=w432) -> (abs(x)=w430:dbl)
        n189 = Absolute Value(x=w431) -> (abs(x)=w428:dbl)
        n190 = Not Equal To 0?(x=w428) -> (x != 0?=w429:bool)
        n191 = Unbundle By Name(w386) -> ("DLTS properties.Instant start"=w390:bool)
        n192 = case shown="True" w429 {
          tunnel: w430 -> [_ w470]
          tunnel: w428 -> [_ w469]
          tunnel: w418 -> [_ w467]
          tunnel: [FALSE w466] -> w424
          frame False {
          }
          frame True {
            n193 = Divide(x=w470, y=w469) -> (x/y=w468:dbl)
            n194 = Greater?(x=w467, y=w468) -> (0:w466:bool)
          }
        }
        n195 = And(x=w424, y=w423) -> (x .and. y?=w392:bool)
        n196 = Unbundle By Name(w386) -> ("DLTS properties.Tstop"=w393:dbl[unit], "DLTS properties.T rate"=w394:dbl[unit])
        n197 = Unbundle By Name(w402) -> ("Temp handle"=w401:T5)
        n198 = Compound Arithmetic op=OR(w392, w391, w390) -> (w389:bool)
        n199 = case shown="True" w389 {
          tunnel: [cluster{"Data":variant, "Message":string} {"Data"=variant, "Message"="Wait_temp"} ("element") cluster{"Data":variant, "Message":string} {"Data"=variant, "Message"="Measure"} ("element")] -> w411
          tunnel: [w435 w450] -> w407
          tunnel: w406 -> [w435 w446]
          tunnel: w405 -> [_ w452]
          tunnel: w403 -> [_ w448]
          tunnel: w401 -> [_ w438]
          tunnel: w400 -> [_ w443]
          tunnel: w394 -> [_ w442]
          tunnel: w393 -> [_ w441]
          frame False {
            # "Temperature not reached, repeat Wait_temp step"
            n200 = Wait (ms)(milliseconds to wait=u32 4500) -> ()  [unwired: 1 out]
          }
          frame True {
            # "Enable MFIA's output"
            # "Update progress bar"
            # "Start temperature ramp"
            # "Temperature reached (or Instant start is On) - start colecting data"
            n201 = call <vilib>:"Acquire Semaphore.vi"("error in (no error)"=w446, "semaphore"=w443) -> ("error out"=w440:errorcluster, "semaphore out"=w444:T29)  [unwired: 3 in, 1 out]
            n202 = call "Temp ctrl - Ramp Setpoint.vi"("Error In"=w440, "Speed"=w442, "Setpoint"=w441, "Temp handle"=w438) -> ("Error Out"=w439:errorcluster)  [unwired: 7 in]
            n203 = call <vilib>:"Release Semaphore.vi"("error in (no error)"=w439, "semaphore"=w444) -> ("error out"=w445:errorcluster)  [unwired: 4 in, 1 out]
            n204 = disable-structure shown="Default" {
              disable-tunnel: w448 -> [w463 _]
              disable-tunnel: [w460 w464] -> w447
              disable-tunnel: w445 -> [w458 w464]
              frame condition #0 (active) {
                w462 = T31 2 items=["NoProgress"=0, "Indeterminate"=1, "Normal"=2, "Error"=4, "Paused"=8] ("State (No Progress)")
                n205 = call <vilib>:"Set Progress State.vi"("error in (no error)"=w458, "State (No Progress)"=w462, "Window Handle"=w463) -> ("error out"=w461:errorcluster, "dup Window Handle"=w459:refnum<k24>)  [unwired: 7 in]
                n206 = call <vilib>:"Set Progress Value.vi"("error in (no error)"=w461, "Window Handle"=w459) -> ("error out"=w460:errorcluster)  [unwired: 8 in, 1 out]
              }
              frame condition #1 {
              }
            }
            n207 = Boolean To (0,1)(Boolean=TRUE) -> (0, 1=w456:i16)
            n208 = call-poly <instrlib>:"ziSetValue.vi"("Error In"=w447, "Value"=w456, "Path"="imps/0/output/on", "Handle In"=w452) -> ("Error Out"=w451:errorcluster)  [unwired: 1 in, 1 out]
            n209 = Wait (ms)(milliseconds to wait=u32 1000) -> ()  [unwired: 1 out]
            n210 = property on="Measurement info" class="Str"(error in=w451, "Value"="Starting data acquisition" ("Measurement info")) -> (error out=w450:errorcluster)  [unwired: 1 in, 1 out]
          }
        }
        n211 = Enqueue Element(queue=w412, element=w411, error in (no error)=w407) -> (error out=w404:errorcluster)  [unwired: 1 in, 2 out]
      }
      frame "Measure" {
        # "Update GUI"
        # "Enqueue next step of measurement"
        # "Enqueue data to the Analysis Handling Loop"
        # "Measure T"
        # "Measure  C(t)"
        # "Capture transient and temperature -> send to AHL; calculate progress -> repeat or finalize measurement"
        n212 = Unbundle By Name(w526) -> ("MFIA handle.ziModHandle"=w528:T20, "MFIA handle.ziHandle"=w527:T19)
        n213 = Unbundle By Name(w498) -> ("DLTS properties.Vpulse"=w489:dbl[unit], "DLTS properties.pulse length"=w486:dbl[unit], "DLTS properties.Pulse 2"=w491:bool, "DLTS properties.pulse length 2"=w490:dbl[unit], "DLTS properties.Vpulse 2"=w488:dbl[unit], "DLTS properties.Vbias"=w487:dbl[unit], "DLTS properties.Averaging"=w485:dbl)
        n214 = case shown="True" w491 {
          tunnel: w529 -> [w536 w549]
          tunnel: w528 -> [w535 w547]
          tunnel: w527 -> [w534 w548]
          tunnel: [w533 w543] -> w525
          tunnel: [w532 w546] -> w497
          tunnel: [w531 w545] -> w496
          tunnel: [w530 w544] -> w495
          tunnel: w490 -> [_ w539]
          tunnel: w489 -> [_ w542]
          tunnel: w488 -> [_ w538]
          tunnel: w487 -> [_ w537]
          tunnel: w486 -> [_ w541]
          tunnel: w485 -> [_ w540]
          frame False {
            n215 = call "DLTS - run DAQ (SubVI).vi"("error in (no error)"=w536, "Handle in"=w534, "ModHandle in"=w535) -> ("error out"=w532:errorcluster, "t"=w531:dbl[], "Samples"=w530:dbl[], "ModHandle Out  out"=w533:T20)  [unwired: 4 in, 1 out]
          }
          frame True {
            n216 = call "DLTS - run 2 pulse DAQ (SubVI).vi"("ziModHandle"=w547, "ziHandle"=w548, "pulse length 2"=w539, "Vpulse 2"=w538, "Vbias"=w537, "error in (no error)"=w549, "pulse length"=w541, "Vpulse"=w542, "Averaging"=w540) -> ("ModHandle Out"=w543:T20, "t"=w545:dbl[], "Capacitance transient"=w544:dbl[], "error out"=w546:errorcluster)  [unwired: 7 in]
          }
        }
        n217 = Bundle By Name(cluster=w526, "MFIA handle.ziModHandle"=w525) -> (w523:T3)
        n218 = Unbundle By Name(w498) -> ("Settings.Temp ctrl.Stabilization rate"=w479:dbl, "DLTS properties.Tstart"=w517:dbl[unit], "DLTS properties.Tstop"=w482:dbl[unit], "DLTS properties.Emission rate"=w518:dbl[unit][], "Settings.Temp ctrl.Stabilization delta"=w477:dbl)
        n219 = Bundle("t"=w496, "Capacitance transient"=w495) -> (→"Transient Graph":T32)  [unwired: 1 in]
        n220 = Unbundle By Name(w523) -> ("Temp handle"=w494:T5)
        n221 = call <vilib>:"Acquire Semaphore.vi"("error in (no error)"=w497, "semaphore"=w522) -> ("error out"=w493:errorcluster, "semaphore out"=w524:T29)  [unwired: 3 in, 1 out]
        n222 = call "Temp ctrl - Read temp and stp.vi"("Error In"=w493, "Temp handle"=w494) -> ("Error Out"=w492:errorcluster, "Sample temperature"=w481:dbl[unit])  [unwired: 2 in, 3 out]
        n223 = call <vilib>:"Release Semaphore.vi"("error in (no error)"=w492, "semaphore"=w524) -> ("error out"=w521:errorcluster)  [unwired: 4 in, 1 out]
        n224 = Subtract(x=w482, y=w481) -> (x-y=w480:dbl[unit])
        n225 = Absolute Value(x=w480) -> (abs(x)=w478:dbl[unit])
        n226 = node(w495) -> (w504:dbl[unit][])
        n227 = node(w496) -> (w503:dbl[unit][])
        n228 = node(w478) -> (w476:dbl)
        n229 = Greater?(x=w476, y=w477) -> (0:w474:bool)
        n230 = call "cDLTS temperature not stable.vi"("Stabilization rate"=w479, "Current sample temperature"=w481, "Temperature history in"=w483) -> ("Temperature not stable"=w475:bool, "Temperature history out"=w484:T23)  [unwired: 7 in]
        n231 = call "cDLTS progress.vi"("Current sample temperature"=w481, "Tstop"=w482, "Tstart"=w517) -> ("Progress"=w507:dbl, "Still not finished"=w472:bool)  [unwired: 7 in]
        n232 = Or(x=w475, y=w474) -> (x .or. y?=w473:bool)
        n233 = And(x=w472, y=w473) -> (x .and. y?=w471:bool)
        n234 = Unbundle By Name(w498) -> ("actual t_w"=w500:dbl[unit][], "R_peak"=w499:dbl[])
        n235 = Bundle By Name(cluster=T27 {"Message"="", "C(t)"=[], "t"=[], "tau"=[], "T"=0.0, "actual t_w"=[], "R_peak"=[]} ("element"), "actual t_w"=w500, "R_peak"=w499, "Message"="Analyze", "tau"=w518, "T"=w481, "C(t)"=w504, "t"=w503) -> (w502:T27)
        n236 = Enqueue Element(queue=w520, element=w502, error in (no error)=w521) -> (error out=w516:errorcluster)  [unwired: 1 in, 2 out]
        n237 = Select(t=cluster{"Data":variant, "Message":string} {"Data"=variant, "Message"="Measure"}, s=w471, f=cluster{"Data":variant, "Message":string} {"Data"=variant, "Message"="Finalize"}) -> (s? t:f=w513:cluster{"Data":variant, "Message":string})
        n238 = Enqueue Element(queue=w512, element=w513, error in (no error)=w516) -> (error out=w506:errorcluster)  [unwired: 1 in, 2 out]
        n239 = case shown="True" w471 {
          tunnel: [w552 w565] -> w510
          tunnel: ["Finalizing" w564] -> w509
          tunnel: w507 -> [_ w561]
          tunnel: w506 -> [w551 w562]
          tunnel: w505 -> [w550 w560]
          frame False {
            n240 = disable-structure shown="Default" {
              disable-tunnel: [w557 w558] -> w552
              disable-tunnel: w551 -> [w556 w558]
              disable-tunnel: w550 -> [w554 _]
              frame condition #0 (active) {
                w555 = T31 1 items=["NoProgress"=0, "Indeterminate"=1, "Normal"=2, "Error"=4, "Paused"=8] ("State (No Progress)")
                n241 = call <vilib>:"Set Progress State.vi"("error in (no error)"=w556, "State (No Progress)"=w555, "Window Handle"=w554) -> ("error out"=w557:errorcluster)  [unwired: 7 in, 1 out]
              }
              frame condition #1 {
              }
            }
          }
          frame True {
            n242 = disable-structure shown="TARGET_TYPE==Windows" {
              disable-tunnel: w562 -> [w569 w570]
              disable-tunnel: w561 -> [w568 _]
              disable-tunnel: w560 -> [w567 _]
              disable-tunnel: [w566 w570] -> w559
              frame condition #0 (active) {
                n243 = call <vilib>:"Set Progress Value.vi"("error in (no error)"=w569, "current (0)"=w568, "Window Handle"=w567) -> ("error out"=w566:errorcluster)  [unwired: 7 in, 1 out]
              }
              frame condition #1 {
              }
            }
            n244 = Format Into String(format string="Measurement in progress \\n%d %%", error in=w559, w561) -> (resulting string=w564:string, error out=w565:errorcluster)  [unwired: 1 in]
          }
        }
        n245 = property on="Measurement info" class="Str"(error in=w510, "Value"=w509) -> (error out=w511:errorcluster)  [unwired: 1 in, 1 out]
      }
      frame "Finalize" {
        w583 = T28."Enabled" ("Disabled")
        # "Reset MFIA's parameters"
        # "Reset temperature ramp\n(current reading as setpoint)"
        # "Enqueue \"Save\" in \nAnalysis Handling Loop"
        # "Reset temperature controler and MFIA, save results and update Front Panel"
        n246 = Unbundle By Name(w594) -> ("MFIA handle.ziHandle"=w595:T19, "MFIA handle.ziModHandle"=w573:T20, "Temp handle"=w589:T5)
        n247 = Enqueue Element(queue=w605, element=T27 {"Message"="Save", "C(t)"=[], "t"=[], "tau"=[], "T"=0.0, "actual t_w"=[], "R_peak"=[]}, error in (no error)=w606) -> (error out=w603:errorcluster)  [unwired: 1 in, 2 out]
        n248 = call <vilib>:"Acquire Semaphore.vi"("error in (no error)"=w603, "semaphore"=w602) -> ("error out"=w588:errorcluster, "semaphore out"=w604:T29)  [unwired: 3 in, 1 out]
        n249 = call "Temp ctrl - Disable Ramp.vi"("Error In"=w588, "Temp handle"=w589) -> ("Error Out"=w591:errorcluster)  [unwired: 9 in]
        n250 = call "Temp ctrl - Read temp and stp.vi"("Error In"=w591, "Temp handle"=w589) -> ("Error Out"=w590:errorcluster, "Sample temperature"=w578:dbl[unit])  [unwired: 2 in, 3 out]
        n251 = Select(t="Post meas. temp.", s="Enable post meas. T", f=w578) -> (s? t:f=w580:dbl[unit])
        n252 = call "Temp ctrl - Setpoint.vi"("Error In"=w590, "Setpoint"=w580, "Temp handle"=w589) -> ("Error Out"=w587:errorcluster)  [unwired: 8 in]
        n253 = call <vilib>:"Release Semaphore.vi"("error in (no error)"=w587, "semaphore"=w604) -> ("error out"=w600:errorcluster)  [unwired: 4 in, 1 out]
        n254 = call "DLTS - reset bias (SubVI).vi"("error in (no error)"=w600, "Handle in"=w595) -> ("error out"=w599:errorcluster, "Handle out"=w598:T19)  [unwired: 8 in]
        n255 = call "DLTS - reset impedance (SubVI).vi"("error in (no error)"=w599, "Handle in"=w598) -> ("error out"=w597:errorcluster, "Handle out"=w596:T19)  [unwired: 8 in]
        n256 = call "DLTS - reset pulse timing (SubVI).vi"("error in (no error)"=w597, "Handle in"=w596) -> ("error out"=w575:errorcluster, "Handle out"=w576:T19)  [unwired: 8 in]
        n257 = call <instrlib>:"ziModClear.vi"("Error In"=w575, "ziModHandle In"=w573) -> ("Error Out"=w574:errorcluster, "ModHandle Out"=w572:T20)  [unwired: 7 in]
        n258 = Bundle By Name(cluster=w594, "MFIA handle.ziHandle"=w576, "MFIA handle.ziModHandle"=w572) -> (w593:T3)
        n259 = property on="Measure" class="Bool"(error in=w574, "DisabledEnum"=w583) -> (error out=w582:errorcluster)  [unwired: 1 in, 1 out]
        n260 = property on="Setpoint" class="DigNum (strict)"(error in=w582, "DisabledEnum"=w583) -> (error out=w581:errorcluster)  [unwired: 1 in, 1 out]
        n261 = property on="Measurement info" class="Str"(error in=w581, "Value"="Done!" ("Measurement info")) -> (error out=w585:errorcluster)  [unwired: 1 in, 1 out]
        n262 = disable-structure shown="Default" {
          disable-tunnel: w607 -> [w612 _]
          disable-tunnel: [w609 w613] -> w586
          disable-tunnel: w585 -> [w608 w613]
          frame condition #0 (active) {
            n263 = call <vilib>:"Set Progress Value.vi"("error in (no error)"=w608, "Window Handle"=w612) -> ("error out"=w610:errorcluster, "dup Window Handle"=w611:refnum<k24>)  [unwired: 8 in]
            n264 = call <vilib>:"Set Progress State.vi"("error in (no error)"=w610, "Window Handle"=w611) -> ("error out"=w609:errorcluster)  [unwired: 8 in, 1 out]
          }
          frame condition #1 {
          }
        }
      }
      frame "Abort" {
        # "Remove queued control messages and set MHL to \"Finalize\""
        n265 = disable-structure shown="Default" {
          disable-tunnel: w617 -> [w633 w635]
          disable-tunnel: [w632 w635] -> w616
          disable-tunnel: w615 -> [w631 _]
          frame condition #0 (active) {
            w634 = T31 1 items=["NoProgress"=0, "Indeterminate"=1, "Normal"=2, "Error"=4, "Paused"=8] ("State (No Progress)")
            n266 = call <vilib>:"Set Progress State.vi"("error in (no error)"=w633, "State (No Progress)"=w634, "Window Handle"=w631) -> ("error out"=w632:errorcluster)  [unwired: 7 in, 1 out]
          }
          frame condition #1 {
          }
        }
        n267 = Flush Queue(queue=w628, error in (no error)=w616) -> (queue out=w622:refnum<queue>, remaining elements=w623:cluster{"Data":variant, "Message":string}[], error out=w621:errorcluster)
        n268 = for {
          tunnel: w623 -> [w636] mode=indexing
          tunnel: w622 -> [w641]
          tunnel: w621 -> [w642]
          tunnel: string[] ["Measure", "Prepare", "Wait_temp", "Finalize"] ("1D array") -> [w639]
          tunnel: [w638] -> w619
          tunnel: [w637] -> w618
          n269 = Unbundle By Name(w636) -> ("Message"=w643:string)
          n270 = Search 1D Array(1D array=w639, element=w643) -> (index of element=w640:i32)  [unwired: 1 in]
          n271 = case shown="-1" w640 {
            tunnel: w642 -> [w644 w650]
            tunnel: w641 -> [w645 w649]
            tunnel: [w645 w648] -> w638
            tunnel: [w644 w647] -> w637
            tunnel: w636 -> [_ w646]
            frame 0, Default {
            }
            frame -1 {
              n272 = Enqueue Element(queue=w649, element=w646, error in (no error)=w650) -> (queue out=w648:refnum<queue>, error out=w647:errorcluster)  [unwired: 1 in, 1 out]
            }
          }
        }
        n273 = Enqueue Element At Opposite End(queue=w619, element=cluster{"Data":variant, "Message":string} {"Data"=variant, "Message"="Finalize"}, error in (no error)=w618) -> (error out=w624:errorcluster)  [unwired: 1 in, 2 out]
        n274 = property on="Measurement info" class="Str"(error in=w624, "Value"="Measurement aborted" ("Measurement info")) -> (error out=w627:errorcluster)  [unwired: 1 in, 1 out]
      }
      frame "Stop" {
        # "Stop AHL and this loop"
        n275 = Generate User Event(user event=w660, event data cluster=TRUE ("event data"), error in=w661) -> (error out=w655:errorcluster)  [unwired: 1 in, 1 out]
        n276 = Enqueue Element(queue=w653, element=T27 {"Message"="Stop", "C(t)"=[], "t"=[], "tau"=[], "T"=0.0, "actual t_w"=[], "R_peak"=[]}, error in (no error)=w655) -> (error out=w654:errorcluster)  [unwired: 1 in, 2 out]
      }
    }
    n277 = call <vilib>:"General Error Handler.vi"("type of dialog (OK msg:1)"=w271, "error in (no error)"=w272) -> ("error out"=w273:errorcluster)  [unwired: 9 in, 4 out]
    n278 = call <vilib>:"Clear Errors.vi"("error in (no error)"=w273) -> ("error out"=w269:errorcluster)  [unwired: 5 in, 1 out]
  }
  n279 = while "Event Handling Loop" {
    shift-right: [w677] -> w129
    shift-left: w22 -> [w680]
    shift-right: [w678] -> w90
    shift-left: "cDLTS measurement" -> [w679]
    shift-right: [w664] -> w107
    shift-left: w65 -> [w681]
    tunnel: w105 -> [w676]
    tunnel: w122 -> [w675]
    tunnel: [w674] -> w106
    shift-right: [w672] -> w99
    shift-left: FALSE -> [w673]
    tunnel: w69 -> [w671]
    tunnel: w59 -> [w670]
    tunnel: "Session properties" -> [w665]
    tunnel: w19 -> [w663]
    tunnel: w11 -> [w662]
    stop <- w682 stop-if-true
    w666 = T30 2 items=["no dialog", "OK message", "continue or stop message", "OK message + warnings", "continue/stop + warnings"] ("type of dialog (OK msg:1)")
    # "Event Handling Loop"
    n280 = event shown="[9] \"Measure\": Value Change" {
      selector: w675 -> [_ _ _ _ _ _ _ _ _ _ _ _ _ _ _ _]
      dyn-events: [_ _ _ _ _ _ _ _ _ _ _ _ _ _ _ _] -> w674
      timeout: 1000 -> [_ _ _ _ _ _ _ _ _ _ _ _ _ _ _ _]
      tunnel: [_ w711 _ _ _ _ _ _ _ _ _ _ _ _ _ _] -> w682
      tunnel: w681 -> [w689 w717 w741 w751 w762 w771 w785 w804 w817 w857 w909 w916 w946 w978 w991 w1023]
      tunnel: w680 -> [w685 w723 w738 w754 w759 w768 w783 w807 w816 w889 w910 w926 w950 w986 w994 w1022]
      tunnel: w679 -> [w690 w724 w739 w757 w760 w769 w784 w806 w815 w876 w911 w927 w949 w980 w993 w1026]
      tunnel: [w690 w724 w739 w757 w760 w769 w784 w806 w815 w875 w911 w927 w948 w980 w989 w1026] -> w678
      tunnel: [w685 w723 w738 w754 w759 w768 w783 w807 w816 w889 w910 w926 w950 w986 w994 w1022] -> w677
      tunnel: [w688 w722 w740 w748 w761 w770 w776 w789 w812 w885 w909 w915 w945 w983 w990 w1027] -> w667
      tunnel: w676 -> [_ w720 _ _ _ _ _ _ _ w883 _ _ _ w982 _ _]
      tunnel: w673 -> [w687 w721 w737 w756 w758 w767 w782 w805 w814 _ w908 w925 w943 w976 w988 w1028]
      tunnel: [w687 w721 w737 w756 w758 w767 w782 w805 w814 TRUE w908 w925 w947 w976 w987 w1028] -> w672
      tunnel: w671 -> [w686 _ _ w752 _ _ _ _ _ _ _ _ _ _ _ _]
      tunnel: w670 -> [_ _ _ _ _ _ _ _ _ _ _ _ _ _ _ _]
      tunnel: w665 -> [_ _ _ _ _ _ _ _ _ _ _ _ _ _ _ w1025]
      tunnel: w663 -> [_ w715 _ _ _ _ _ _ _ _ _ _ _ _ _ _]
      tunnel: w662 -> [_ _ _ _ _ _ w778 _ w811 _ _ _ _ _ _ _]
      event Timeout {
        # "Refresh temperature and setpoint reading on Front Panel"
        n281 = event-data() -> ()  [unwired: 1 in, 1 out]
        n282 = Unbundle By Name(w685) -> ("Temp handle"=w684:T5, "Temp handle.Connected"=w683:bool)
        n283 = case shown="True" w683 {
          tunnel: w689 -> [w691 w705]
          tunnel: [w691 w704] -> w688
          tunnel: w686 -> [_ w703]
          tunnel: w684 -> [_ w698]
          frame False {
          }
          frame True {
            n284 = local read "Instant T start"() -> (w699:bool)
            n285 = call <vilib>:"Acquire Semaphore.vi"("error in (no error)"=w705, "semaphore"=w703) -> ("error out"=w697:errorcluster, "semaphore out"=w700:T29)  [unwired: 3 in, 1 out]
            n286 = call "Temp ctrl - Read temp and stp.vi"("Error In"=w697, "Temp handle"=w698) -> ("Error Out"=w693:errorcluster, "Sample temperature"=w696:dbl[unit], "Setpoint"=w692:dbl[unit])  [unwired: 2 in, 2 out]
            "Temperature" <- w696
            n287 = case shown="True" w699 {
              tunnel: w696 -> [_ w706]
              frame False {
              }
              frame True {
                n288 = local write "Start temp."(w706) -> ()
              }
            }
            n289 = Cast Unit Bases(0:w696) -> (2:→"Temp Chart":dbl)  [unwired: 1 in]
            n290 = property on="Setpoint" class="DigNum (strict)"(error in=w693) -> (error out=w702:errorcluster, "Key Focus"=w694:bool)  [unwired: 1 in, 1 out]
            n291 = case shown="False" w694 {
              tunnel: w702 -> [w708 w710]
              tunnel: [w709 w710] -> w701
              tunnel: w692 -> [w707 _]
              frame False {
                # "Update setpoint if not currently edited"
                n292 = property on="Setpoint" class="DigNum (strict)"(error in=w708, "Value"=w707) -> (error out=w709:errorcluster)  [unwired: 1 in, 1 out]
              }
              frame True {
              }
            }
            n293 = call <vilib>:"Release Semaphore.vi"("error in (no error)"=w701, "semaphore"=w700) -> ("error out"=w704:errorcluster)  [unwired: 4 in, 1 out]
          }
        }
      }
      event Panel Close? {
        # "Check whether measurement and analysis are finished: if yes stop the loop, if no display dialog"
        n294 = event-data() -> ()  [unwired: 1 in, 1 out]
        n295 = Get Queue Status(queue=w715, error in (no error)=w717) -> (error out=w716:errorcluster, # elements in queue=w713:i32)  [unwired: 1 in, 6 out]
        n296 = Get Queue Status(queue=w720, error in (no error)=w716) -> (queue out=w719:refnum<queue>, error out=w718:errorcluster, # elements in queue=w714:i32)  [unwired: 1 in, 5 out]
        n297 = Add(x=w714, y=w713) -> (x+y=w712:i32)
        n298 = case shown="1, Default" w712 {
          tunnel: [w728 w732] -> w722
          tunnel: w719 -> [_ w731]
          tunnel: w718 -> [w728 w730]
          tunnel: [FALSE TRUE] -> w711
          frame 1, Default {
            n299 = One Button Dialog(message="A measurement is still running.\nWait until it completes or or stop it manually before closing this window") -> ()  [unwired: 1 in, 1 out]
          }
          frame 0 {
            n300 = Bundle By Name(cluster=cluster{"Data":variant, "Message":string} {"Data"=variant, "Message"=""}, "Message"="Stop") -> (w734:cluster{"Data":variant, "Message":string})
            n301 = Enqueue Element(queue=w731, element=w734, error in (no error)=w730) -> (error out=w732:errorcluster)  [unwired: 1 in, 2 out]
          }
        }
        n302 = event-data("Discard?"=TRUE) -> ()  [unwired: 1 in, 1 out]
      }
      event "Top Buttons.Help": Value Change {
        n303 = event-data() -> ("NewVal"=w736:bool)  [unwired: 1 in]
        n304 = case shown="True" w736 {
          tunnel: w741 -> [w742 w746]
          tunnel: [w742 w745] -> w740
          tunnel: w738 -> [_ w744]
          frame False {
          }
          frame True {
            n305 = Unbundle By Name(w744) -> ("Paths.Manual"=w743:path)
            n306 = call "OpenDoc Browser.vi"("error in (no error)"=w746, "File"=w743) -> ("error out"=w745:errorcluster)  [unwired: 9 in]
          }
        }
      }
      event "Setpoint": Value Change {
        # "Update temperature setpoint"
        n307 = event-data() -> ()  [unwired: 1 in, 1 out]
        n308 = call <vilib>:"Acquire Semaphore.vi"("error in (no error)"=w751, "semaphore"=w752) -> ("error out"=w750:errorcluster, "semaphore out"=w747:T29)  [unwired: 3 in, 1 out]
        n309 = Unbundle By Name(w754) -> ("Temp handle"=w753:T5)
        n310 = call "Temp ctrl - Setpoint.vi"("Error In"=w750, "Setpoint"="Setpoint", "Temp handle"=w753) -> ("Error Out"=w749:errorcluster)  [unwired: 8 in]
        n311 = call <vilib>:"Release Semaphore.vi"("error in (no error)"=w749, "semaphore"=w747) -> ("error out"=w748:errorcluster)  [unwired: 4 in, 1 out]
      }
      event "Instant T start": Value Change {
        # "Format Start temp. control"
        n312 = event-data() -> ("NewVal"=w763:bool)  [unwired: 1 in]
        n313 = Select(t=T28."Disabled and Grayed Out", s=w763, f=T28."Enabled") -> (s? t:f=w766:T28)
        n314 = property on="Start temp." class="DigNum (strict)"(error in=w762, "DisabledEnum"=w766) -> (error out=w761:errorcluster)  [unwired: 1 in, 1 out]
      }
      event "Enable post meas. T": Value Change {
        # "Format Start temp. control"
        n315 = event-data() -> ("NewVal"=w772:bool)  [unwired: 1 in]
        n316 = Select(t=T28."Enabled", s=w772, f=T28."Disabled and Grayed Out") -> (s? t:f=w775:T28)
        n317 = property on="Post meas. temp." class="DigNum (strict)"(error in=w771, "DisabledEnum"=w775) -> (error out=w770:errorcluster)  [unwired: 1 in, 1 out]
      }
      event "2nd pulse": Value Change {
        # "Format 2nd pulse controls"
        n318 = event-data() -> ("NewVal"=w786:bool)  [unwired: 1 in]
        n319 = Select(t=T28."Enabled", s=w786, f=T28."Disabled and Grayed Out") -> (s? t:f=w781:T28)
        n320 = property on="2nd pulse length" class="DigNum (strict)"(error in=w785, "DisabledEnum"=w781) -> (error out=w780:errorcluster)  [unwired: 1 in, 1 out]
        n321 = property on="2nd pulse voltage" class="DigNum (strict)"(error in=w780, "DisabledEnum"=w781) -> (error out=w777:errorcluster)  [unwired: 1 in, 1 out]
        n322 = Generate User Event(user event=w778, event data cluster=0.0 ("event data"), error in=w777) -> (error out=w776:errorcluster)  [unwired: 1 in, 1 out]
      }
      event "Rate windows", "Averaging", "Sampling rate", "Acquisition delay": Value Change; User Event {
        # "Recalculate measurement time and number of samples"
        n323 = event-data() -> ()  [unwired: 1 in, 1 out]
        n324 = local read "Rate windows"() -> (w802:dbl[unit][])
        n325 = local read "Sampling rate"() -> (w801:dbl)
        n326 = local read "Averaging"() -> (w800:dbl)
        n327 = local read "1st pulse length"() -> (w799:dbl[unit])
        n328 = local read "2nd pulse length"() -> (w798:dbl[unit])
        n329 = local read "Acquisition delay"() -> (w797:dbl[unit])
        n330 = local read "2nd pulse"() -> (w796:bool)
        n331 = call-poly "DLTS - timing calculation (SubVI).vi"("Emission rates"=w802, "Sampling rate"=w801, "Averaging"=w800, "1st pulse duration"=w799, "2nd Pulse duration"=w798, "Acquisition delay"=w797, "2 pulse mode"=w796) -> ("Number of samples"=w795:i32, "Acquisition duration"=w794:dbl[unit])  [unwired: 10 in, 1 out]
        n332 = property on="No samples" class="DigNum (strict)"(error in=w804, "Val(Sgnl)"=w795) -> (error out=w803:errorcluster)  [unwired: 1 in, 1 out]
        n333 = Greater?(x=w794, y=dbl[unit] 30.0) -> (0:w792:bool)
        n334 = property on="Single transient capture duration" class="DigNum (strict)"(error in=w803, "Val(Sgnl)"=w794) -> (error out=w790:errorcluster)  [unwired: 1 in, 1 out]
        n335 = case shown="False" w792 {
          tunnel: [u32 16777216 ("Numeric Text.Colors:BG Color") u32 16676473 ("Numeric Text.Colors:BG Color")] -> w791
          frame False {
          }
          frame True {
          }
        }
        n336 = property on="Single transient capture duration" class="DigNum (strict)"(error in=w790, "NumText.BG Color"=w791) -> (error out=w789:errorcluster)  [unwired: 1 in, 1 out]
      }
      event "1st pulse length", "2nd pulse length": Value Change {
        w821 = dbl[unit] 2.333e-07  # s
        # "Coerce length of the filling pulse to values available in MFIA"
        n337 = event-data() -> ("CtlRef"=w820:refnum<vi>, "NewVal"=w818:dbl[unit])  [unwired: 1 in]
        n338 = Divide(x=w818, y=w821) -> (x/y=w823:dbl)
        n339 = Round To Nearest(number=w823) -> (nearest integer value=w822:dbl)
        n340 = Multiply(x=w822, y=w821) -> (x*y=w819:dbl[unit])
        n341 = property class="DigNum (strict)"(reference=w820, error in=w817, "Value"=w819) -> (error out=w813:errorcluster)  [unwired: 1 out]
        n342 = Generate User Event(user event=w811, event data cluster=0.0 ("event data"), error in=w813) -> (error out=w812:errorcluster)  [unwired: 1 in, 1 out]
      }
      event "Measure": Value Change {
        w845 = FALSE ("Visible")
        w854 = 5 ("y")
        w843 = T28."Disabled and Grayed Out" ("Disabled")
        # "Rename folder"
        # "New Folder"
        # "Old Folder"
        # "Send Settings and DLTS params to MHL"
        # "Update legend strings"
        # "Clear plot and resize legend"
        # "Flag measurement as \"modified\""
        # "Prepare Front Panel (incl. plots) for a measurement, trigger Measurement Handling Loop"
        n343 = event-data() -> ()  [unwired: 1 in, 1 out]
        n344 = property on="Save Parameters" class="Bool (strict)"(error in=w857, "Visible"=w845) -> (error out=w844:errorcluster)  [unwired: 1 in, 1 out]
        n345 = property on="Export" class="Bool"(error in=w844, "Visible"=w845) -> (error out=w842:errorcluster)  [unwired: 1 in, 1 out]
        n346 = node("Sampling rate") -> (w851:dbl[unit])
        n347 = Unbundle By Name(w876) -> ("Folder"=w831:path, "DLTS properties"=w882:T16)
        n348 = Bundle By Name(cluster=w882, "Tstart"="Start temp.", "Tstop"="Stop temp.", "T rate"="T rate", "Averaging"="Averaging", "I range"="I range", "Test signal"="Test signal", "V range"="V range", "Test frequency"="Test frequency", "Vbias"="Bias voltage", "Vpulse"="1st pulse voltage", "pulse length"="1st pulse length", "Emission rate"="Rate windows", "Sampling rate"=w851, "Bandwidth"="Filter bandwidth", "Pulse 2"="2nd pulse", "Vpulse 2"="2nd pulse voltage", "pulse length 2"="2nd pulse length", "Acq. delay"="Acquisition delay", "Instant start"="Instant T start", "Filter order"="Filter order", "Equivalent circuit model"="Model") -> (w833:T16)
        n349 = property on="Setpoint" class="DigNum (strict)"(error in=w842, "DisabledEnum"=w843) -> (error out=w841:errorcluster)  [unwired: 1 in, 1 out]
        n350 = property on="Measure" class="Bool"(error in=w841, "DisabledEnum"=w843) -> (error out=w858:errorcluster)  [unwired: 1 in, 1 out]
        n351 = call "myDLTS GUID.vi"() -> ("GUID"=w826:string)  [unwired: 1 in]
        n352 = Strip Path(path=w831) -> (stripped path=w839:path)  [unwired: 1 out]
        n353 = local read "Workspace"() -> (w830:path)
        n354 = Array Size(array="Rate windows") -> (size(s)=w860:i32)
        n355 = Build Path(base path=w839, name or relative path=w826) -> (appended path=w829:path)
        n356 = Less?(x=w860, y=w854) -> (x < y?=w863:bool)
        n357 = Build Path(base path=w830, name or relative path=w831) -> (appended path=w828:path)
        n358 = Select(t=w860, s=w863, f=w854) -> (s? t:f=w861:i32)
        n359 = Not(x=w863) -> (.not. x?=w862:bool)
        n360 = Get Date/Time In Seconds() -> (seconds since 1Jan1904=w827:timestamp)
        n361 = Build Path(base path=w830, name or relative path=w829) -> (appended path=w832:path)
        n362 = property on="DLTS Signal Graph" class="XYGraph (strict)"(error in=w858, "LegPlotMin"=w860, "LegNumRows"=w861, "LegScrollVis"=w862, "Value"=cluster{"2D data":dbl[], "2D data":dbl[]}[] [], "LegScrollPos"=u32 0 ("Legend:Scroll Position")) -> (error out=w859:errorcluster)  [unwired: 1 in, 1 out]
        n363 = local write "Folder"(w829) -> ()
        n364 = Bundle By Name(cluster=w876, "GUID"=w826, "Time"=w827, "Folder"=w829, "DLTS properties"=w833) -> (w875:T22)
        n365 = for {
          tunnel: w859 -> [w900]
          tunnel: "Rate windows" -> [w899] mode=indexing
          tunnel: [w898] -> w835
          i -> [w903]
          n366 = Format Into String(format string="Emission Rate = %d 1/s", error in=w900, w899) -> (resulting string=w902:string, error out=w901:errorcluster)  [unwired: 1 in]
          n367 = property on="DLTS Signal Graph" class="XYGraph (strict)"(error in=w901, "Active Plot"=w903, "Plot.Plot Name"=w902, "Plot.Visible?"=TRUE ("Plot.Visible")) -> (error out=w898:errorcluster)  [unwired: 1 in, 1 out]
        }
        n368 = Unbundle By Name(w889) -> ("Settings"=w888:T9)
        n369 = Bundle By Name(cluster=cluster{"Settings":T9, "DLTS properties":T16} {"Settings"={"MFIA"={"Address"="", "Use compensation"=TRUE, "Shut down gracefully"=FALSE}, "Temp ctrl"={"Gain (P)"=0.0, "Reset (I)"=0.0, "Rate (D)"=0.0, "Stabilization rate"=0.0, "Stabilization delta"=0.0, "Type"=enum."Lake Shore 325", "Custom temp ctrl"={"VISA resource name"=""}, "Lakeshore 325"={"VISA name"="", "Loop"=0, "Heater Range"=1, "Heater Resistance"=0, "Sample sensor"=0, "Fast sensor"=0, "Slow sensor"=0}, "Lakeshore 331"={"VISA name"="", "Loop"=1, "Heater Range"=0, "Sample sensor"=0, "Fast sensor"=0, "Slow sensor"=0}, "Lakeshore 332"={"VISA name"="", "Loop"=1, "Heater Range"=0, "Sample sensor"=0, "Fast sensor"=0, "Slow sensor"=0}, "Lakeshore 335"={"VISA name"="", "Loop"=1, "Sample sensor"=0, "Fast sensor"=0, "Slow sensor"=0, "Heater Range"=0, "Output mode"=enum."Off"}, "Lakeshore 336"={"VISA name"="", "Loop"=1, "Output mode"=enum."Off", "Max current"=1.0, "Heater resistance"=1, "Sample sensor"=1, "Slow sensor"=1, "Fast sensor"=1}}, "Source-meter"={"Type"=enum."Custom", "Custom source-meter"={"VISA resource name"=""}, "Keithley 2600"={"VISA name"="", "Ignore ID Query"=FALSE, "SMU"=enum."Channel A"}, "Keithley 2400 Series"={"VISA name"="", "Ignore ID Query"=FALSE}}, "Other"={"Enable OriginLab"=FALSE, "Reader mode"=FALSE, "Auto-save"=FALSE}, "Defaults"={"IV properties"={"T"=0.0, "Vstart"=-0.5, "Vstop"=0.5, "Vpoints"=10.0, "Settling"=0.01, "I limit"=0.1, "Log mapping"=FALSE, "Averaging"=0.0}, "CV properties"={"T"=0.0, "Vstart"=-0.5, "Vstop"=0.5, "Vpoints"=10.0, "Precision"=enum."Normal", "Test signal"=0.01, "Auto I range"=FALSE, "Test frequency"=100000.0, "I range"=-2.0, "V range"=10.0, "Log mapping"=FALSE, "Rel perm"=0.0, "Area"=0.0, "Equivalent circuit model"=0}, "DLTS properties"={"Tstart"=0.0, "Instant start"=FALSE, "Tstop"=0.0, "T rate"=0.0, "Test signal"=0.0, "Test frequency"=0.0, "Bandwidth"=0.0, "Averaging"=0.0, "Vbias"=0.0, "Vpulse"=0.0, "pulse length"=0.0, "Pulse 2"=FALSE, "Vpulse 2"=0.0, "pulse length 2"=0.0, "I range"=-2.0, "V range"=10.0, "Emission rate"=[], "Sampling rate"=0.0, "Acq. delay"=0.0, "Filter order"=0, "Equivalent circuit model"=0}, "LDLTS properties"={"T"=0.0, "Test signal"=0.0, "Test frequency"=0.0, "Bandwidth"=0.0, "Averaging"=0.0, "Vbias"=0.0, "Vpulse"=0.0, "pulse length"=0.0, "Pulse 2"=FALSE, "Vpulse 2"=0.0, "pulse length 2"=0.0, "I range"=-2.0, "V range"=10.0, "Sampling rate"=0.0, "Acq. delay"=0.0, "Sampling time"=0.0, "Filter order"=0, "Equivalent circuit model"=0}}}, "DLTS properties"={"Tstart"=0.0, "Instant start"=FALSE, "Tstop"=0.0, "T rate"=0.0, "Test signal"=0.0, "Test frequency"=0.0, "Bandwidth"=0.0, "Averaging"=0.0, "Vbias"=0.0, "Vpulse"=0.0, "pulse length"=0.0, "Pulse 2"=FALSE, "Vpulse 2"=0.0, "pulse length 2"=0.0, "I range"=-2.0, "V range"=10.0, "Emission rate"=[], "Sampling rate"=0.0, "Acq. delay"=0.0, "Filter order"=0, "Equivalent circuit model"=0}}, "DLTS properties"=w833, "Settings"=w888) -> (w884:cluster{"Settings":T9, "DLTS properties":T16})
        n370 = call <vilib>:"Check if File or Folder Exists.vi"("error in (no error)"=w835, "path"=w828) -> ("error out"=w837:errorcluster, "file or folder exists?"=w838:bool, "dup path"=w836:path)  [unwired: 7 in]
        n371 = case shown="True" w838 {
          tunnel: w836 -> [_ w894]
          tunnel: w832 -> [_ w893]
          tunnel: w837 -> [w890 w892]
          tunnel: [w890 w891] -> w834
          frame False {
          }
          frame True {
            n372 = Move(source path=w894, error in=w892, 9:TRUE ("overwrite (F)"), 10:w893) -> (error out=w891:errorcluster)  [unwired: 1 in, 2 out]
          }
        }
        n373 = Bundle By Name(cluster=cluster{"Data":variant, "Message":string} {"Data"=variant, "Message"=""}, "Data"=w884, "Message"="Prepare") -> (w886:cluster{"Data":variant, "Message":string})
        n374 = property on="Measurement info" class="Str"(error in=w834, "Value"="Progress: 0%" ("Measurement info")) -> (error out=w872:errorcluster)  [unwired: 1 in, 1 out]
        n375 = Enqueue Element(queue=w883, element=w886, error in (no error)=w872) -> (error out=w885:errorcluster)  [unwired: 1 in, 2 out]
      }
      event "Filter bandwidth", "Filter order": Value Change {
        n376 = event-data() -> ()  [unwired: 1 in, 1 out]
        n377 = local read "Filter bandwidth"() -> (w905:dbl[unit])
        n378 = local read "Filter order"() -> (w904:i32)
        n379 = call "MFIA Filter Response Calculation.vi"("Filter order"=w904, "Bandwidth"=w905) -> ("Settling times"=w907:T34)  [unwired: 8 in, 1 out]
        n380 = Unbundle By Name(w907) -> ("T_s 95%"=→"Filter rise time":dbl[unit])
      }
      event "V range", "Test signal", "Bias voltage", "1st pulse voltage", "2nd pulse voltage": Value Change {
        # "Coerce voltages"
        n381 = event-data() -> ()  [unwired: 1 in, 1 out]
        n382 = property on="Test signal" class="DigNum (strict)"(error in=w916) -> (error out=w920:errorcluster, "Value"=w924:dbl[unit])  [unwired: 1 in, 1 out]
        n383 = Multiply(x=w924, y=1.42) -> (x*y=w921:dbl[unit])
        n384 = property on="V range" class="Ring (strict)"(error in=w920) -> (error out=w919:errorcluster, "Value"=w922:dbl[unit])  [unwired: 1 in, 1 out]
        n385 = control-ref of="Bias voltage"() -> (w914:refnum<vi>)
        n386 = control-ref of="1st pulse voltage"() -> (w913:refnum<vi>)
        n387 = control-ref of="2nd pulse voltage"() -> (w912:refnum<vi>)
        n388 = Subtract(x=w922, y=w921) -> (x-y=w918:dbl[unit])
        n389 = Build Array(w914, w913, w912) -> (w917:refnum<vi>[])
        n390 = for {
          tunnel: w919 -> [w932]
          tunnel: w918 -> [w931]
          tunnel: w917 -> [w929] mode=indexing
          tunnel: [w928] -> w915
          n391 = property on="Property Node" class="DigNum (strict)"(reference=w929, error in=w932) -> (reference out=w930:refnum<vi>, error out=w934:errorcluster, "Value"=w933:dbl[unit])
          n392 = Negate(x=w931) -> (-x=w937:dbl[unit])
          n393 = In Range and Coerce(upper limit=w931, x=w933, lower limit=w937) -> (coerced(x)=w935:dbl[unit], In Range?=w936:bool)
          n394 = case shown="False" w936 {
            tunnel: w935 -> [w940 _]
            tunnel: w934 -> [w941 w942]
            tunnel: [w939 w942] -> w928
            tunnel: w930 -> [w938 _]
            frame False {
              # "Coerce"
              n395 = property on="Property Node" class="DigNum (strict)"(reference=w938, error in=w941, "Value"=w940) -> (error out=w939:errorcluster)  [unwired: 1 out]
            }
            frame True {
              # "In Range"
            }
          }
        }
      }
      event "Top Buttons.Save Parameters": Value Change {
        # "Save parameters without triggering the measurement"
        n396 = event-data() -> ("NewVal"=w944:bool)  [unwired: 1 in]
        n397 = case shown="True" w944 {
          tunnel: w949 -> [w953 w974]
          tunnel: [w953 w972] -> w948
          tunnel: [w952 TRUE] -> w947
          tunnel: w946 -> [w951 w969]
          tunnel: [w951 w956] -> w945
          tunnel: w943 -> [w952 _]
          frame False {
          }
          frame True {
            n398 = Unbundle By Name(w974) -> ("DLTS properties"=w975:T16)
            n399 = local read "1st pulse voltage"() -> (w964:dbl[unit])
            n400 = local read "1st pulse length"() -> (w965:dbl[unit])
            n401 = local read "Start temp."() -> (w968:dbl[unit])
            n402 = local read "Stop temp."() -> (w967:dbl[unit])
            n403 = local read "T rate"() -> (w957:dbl[unit])
            n404 = local read "Averaging"() -> (w958:dbl)
            n405 = local read "I range"() -> (w959:dbl)
            n406 = local read "Test signal"() -> (w960:dbl[unit])
            n407 = local read "V range"() -> (w961:dbl[unit])
            n408 = local read "Test frequency"() -> (w962:dbl[unit])
            n409 = local read "Bias voltage"() -> (w963:dbl[unit])
            n410 = local read "Rate windows"() -> (w966:dbl[unit][])
            n411 = local read "Sampling rate"() -> (w955:dbl)
            n412 = node(w955) -> (w954:dbl[unit])
            n413 = Bundle By Name(cluster=w975, "Tstart"=w968, "Tstop"=w967, "T rate"=w957, "Averaging"=w958, "I range"=w959, "Test signal"=w960, "V range"=w961, "Test frequency"=w962, "Vbias"=w963, "Vpulse"=w964, "pulse length"=w965, "Emission rate"=w966, "Sampling rate"=w954) -> (w973:T16)
            n414 = property on="Measurement info" class="Str"(error in=w969, "Value"="Parameters saved" ("Measurement info")) -> (error out=w956:errorcluster)  [unwired: 1 in, 1 out]
            n415 = Bundle By Name(cluster=w974, "DLTS properties"=w973) -> (w972:T22)
          }
        }
      }
      event "Stop": Value Change {
        # "Stop measurement"
        n416 = event-data() -> ()  [unwired: 1 in, 1 out]
        n417 = property on="Stop" class="Bool"(error in=w978, "DisabledEnum"=T28."Disabled and Grayed Out" ("Disabled")) -> (error out=w977:errorcluster)  [unwired: 1 in, 1 out]
        n418 = Bundle By Name(cluster=cluster{"Data":variant, "Message":string} {"Data"=variant, "Message"=""}, "Message"="Abort") -> (w984:cluster{"Data":variant, "Message":string})
        n419 = Enqueue Element At Opposite End(queue=w982, element=w984, error in (no error)=w977) -> (error out=w983:errorcluster)  [unwired: 1 in, 2 out]
      }
      event "Top Buttons.Information": Value Change {
        # "Display Info dialog"
        n420 = event-data() -> ("NewVal"=w992:bool)  [unwired: 1 in]
        n421 = case shown="False" w992 {
          tunnel: w993 -> [w996 w1003]
          tunnel: w991 -> [w995 w1006]
          tunnel: [w995 w1004] -> w990
          tunnel: [w996 w1002] -> w989
          tunnel: w988 -> [w997 w1001]
          tunnel: [w997 w1000] -> w987
          frame False {
          }
          frame True {
            n422 = Unbundle By Name(w1003) -> ("Name"=w1008:string, "Comment"=w1007:string)
            n423 = call "Measurement renamer.vi"("error in (no error)"=w1006, "Comment In"=w1007, "Measurement name In"=w1008) -> ("error out"=w1004:errorcluster, "Canceled"=w1005:bool, "Comment Out"=w998:string, "Measurement name Out"=w999:string)  [unwired: 1 in]
            n424 = case shown="False" w1005 {
              tunnel: w1003 -> [w1012 w1015]
              tunnel: [w1011 w1015] -> w1002
              tunnel: w1001 -> [_ w1014]
              tunnel: [TRUE w1014] -> w1000
              tunnel: w999 -> [w1010 _]
              tunnel: w998 -> [w1009 _]
              frame False {
                n425 = Bundle By Name(cluster=w1012, "Name"=w1010, "Comment"=w1009) -> (w1011:T22)
              }
              frame True {
              }
            }
          }
        }
      }
      event "Top Buttons.Export": Value Change {
        # "Display Export dialog and export data"
        n426 = event-data() -> ()  [unwired: 1 in, 1 out]
        n427 = Unbundle By Name(w1022) -> ("Settings.Other.Enable OriginLab"=w1021:bool)
        n428 = Bundle By Name(cluster=T33 {"Clipboard"=TRUE, "dat"=TRUE, "iso"=FALSE, "Origin"=FALSE, "Excel"=FALSE} ("Available options"), "Origin"=w1021) -> (w1017:T33)
        n429 = local read "Workspace"() -> (w1024:path)
        n430 = call "Export dialog.vi"("error in (no error)"=w1023, "Available options"=w1017) -> ("error out"=w1020:errorcluster, "Option"=w1019:T35)  [unwired: 7 in, 1 out]
        n431 = case shown="\"Clipboard\"" w1019 {
          tunnel: w1020 -> [w1029 w1032 w1038 w1043]
          tunnel: [w1029 w1033 w1035 w1042] -> w1027
          tunnel: w1026 -> [_ w1034 w1036 w1041]
          tunnel: w1025 -> [_ _ _ w1040]
          tunnel: w1024 -> [_ w1031 w1037 w1039]
          tunnel: "myDLTS file path" -> [_ w1030 _ _]
          frame "Canceled", Default {
          }
          frame "Dat" {
            n432 = call-poly "Export single dat - cluster.vi"(".myDLTS file path"=w1030, "Error In"=w1032, "Workspace"=w1031, "cDLTS measurement"=w1034) -> ("Error Out"=w1033:errorcluster)  [unwired: 4 in]
          }
          frame "Clipboard" {
            n433 = call-poly "Export single clipboard - cluster.vi"("Error In"=w1038, "Workspace"=w1037, "cDLTS measurement"=w1036) -> ("Error Out"=w1035:errorcluster)  [unwired: 5 in]
          }
          frame "Origin" {
            n434 = call-poly "Export Origin.vi"("Error In"=w1043, "Workspace"=w1039, "Session properties"=w1040, "cDLTS measurement"=w1041) -> ("Error Out"=w1042:errorcluster)  [unwired: 7 in]
          }
        }
      }
    }
    n435 = call <vilib>:"General Error Handler.vi"("type of dialog (OK msg:1)"=w666, "error in (no error)"=w667) -> ("error out"=w668:errorcluster)  [unwired: 9 in, 4 out]
    n436 = call <vilib>:"Clear Errors.vi"("error in (no error)"=w668) -> ("error out"=w664:errorcluster)  [unwired: 5 in, 1 out]
  }
  "Loop data out" <- w129
  "Modified" <- w99
  "cDLTS measurement out" <- w90
  n437 = Unregister For Events(event registration refnum=w106, error in=w107) -> (error out=w14:errorcluster)
  n438 = Destroy User Event(user event=w11, error in=w14) -> (error out=w13:errorcluster)
  n439 = Destroy User Event(user event=w34, error in=w13) -> (error out=w94:errorcluster)
  n440 = Merge Errors(w94, w92, w62) -> (w93:errorcluster)
  n441 = Release Queue(queue=w105, error in (no error)=w93) -> (error out=w64:errorcluster)  [unwired: 1 in, 2 out]
  n442 = Release Queue(queue=w19, error in (no error)=w64) -> (error out=→"Error Out":errorcluster)  [unwired: 1 in, 2 out]
